vi "Xijk.vi"() -> ()   [LabVIEW 2010]
uses:
  Type Def/filepath.ctl
  Type Def/event.ctl
  Type Def/axis_parameters.ctl
  Type Def/color_parameters.ctl
  Type Def/save_cluster.ctl
  Type Def/configuration_cluster.ctl
  Type Def/search_parameters.ctl
  Type Def/spectra_parameters.ctl
  Type Def/settings.ctl
  Type Def/spectrum_table_control.ctl
  Type Def/xijk_cluster.ctl
  Type Def/control_references_cluster.ctl
  <vilib>/Utility/miscctls.llb/LVPointTypeDef.ctl
  <vilib>/Utility/xml.llb/Write to XML File(string).vi
  subVI/xijk_automatic_read_and_guess.lvlib
  subVI/xijk_select_best_filter.lvlib
  subVI/xijk_combined_file.lvlib
panel:
  in  "Settings":T1={"search parameters"={"Paths"={"Path: Excitation filters"=path "", "Path: Dicroic filters"=path "", "Path: Emission filters"=path "", "Path reget"=path ""}, "table excitation"=[], "table dicroics"=[], "table emission"=[], "Integers"={"Select result number"=1}, "boolean selector array"=[], "table for calculation automagic"=[]}, "output cluster"={"Booleans"={"Unknown detector"=FALSE, "Dual band filters"=FALSE, "Dual emission by cubes"=FALSE, "FRET"=FALSE}, "Integers"={"Light source"=0, "Number of fluorophores"=0, "Wavelength of laser (nm) 1"=0, "Broadness of laser (nm) 1"=0.0, "Wavelength of laser (nm) 2"=0, "Broadness of laser (nm) 2"=0.0, "Template"=1}, "Doubles"={"Molar extinction 1"=1.0, "Molar extinction 2"=1.0, "Quantum efficiency 1"=1.0, "Quantum efficiency 2"=1.0}}, "output cluster 2"={"Excitation filter 1"=path "", "Dichroic filter 1"=path "", "Emission filter 1"=path "", "Excitation filter 2"=path "", "Dichroic filter 2"=path "", "Emission filter 2"=path "", "Extra em filter 1"=path "", "Extra em filter 2"=path "", "Light source file"=path "", "Fluorophore absorption 1"=path "", "Fluorophore emission 1"=path "", "Fluorophore absorption 2"=path "", "Fluorophore emission 2"=path "", "Detector"=path ""}, "cluster de sortie"={"Excitation filter_x"=[], "Excitation filter_y"=[], "Dichroic filter_x"=[], "Dichroic filter_y"=[], "Emission filter_x"=[], "Emission filter_y"=[], "Excitation filter_x 2"=[], "Excitation filter_y 2"=[], "Dichroic filter_x 2"=[], "Dichroic filter_y 2"=[], "Emission filter_x 2"=[], "Emission filter_y 2"=[], "Extra em filter_x 1"=[], "Extra em filter_y 1"=[], "Extra em filter_x 1"=[], "Extra em filter_y 2"=[], "Light source_x"=[], "Light source_y"=[], "Detector_x"=[], "Detector_y"=[], "Fluorophore absorption_x"=[], "Fluorophore absorption_y"=[], "Fluorophore emission_x"=[], "Fluorophore emission_y"=[], "Fluorophore absorption_x 2"=[], "Fluorophore absorption_y 2"=[], "Fluorophore emission_x 2"=[], "Fluorophore emission_y 2"=[], "laser_x"=[], "laser_y"=[], "laser_x 2"=[], "laser_y 2"=[], "quantum efficiency factor 1"=0.0, "quantum efficiency factor 2"=0.0, "lamp scaling factor"=0.0}, "Xijk output cluster"={"Xijk 111"=0.0, "Xijk 112"=0.0, "Xijk 121"=0.0, "Xijk 122"=0.0, "Xijk 211"=0.0, "Xijk 212"=0.0, "Xijk 221"=0.0, "Xijk 222"=0.0, "Eijk 111"=0.0, "Eijk 112"=0.0, "Eijk 121"=0.0, "Eijk 122"=0.0, "Eijk 211"=0.0, "Eijk 212"=0.0, "Eijk 221"=0.0, "Eijk 222"=0.0}, "GUI configuration"={"axes in"={"min x-axis excitation"=300, "max x-axis excitation"=800, "min x-axis emission"=300, "max x-axis emission"=800, "precision of results"=2}, "plot colors in"={"Lanscape Portrait"=FALSE, "Plot logarithmic"=FALSE, "Ex/Em filters double"=FALSE, "Line colors"=[16734569, 56375, 16711916, 5896447, 16448250, 56375]}}, "references"={"Excitation filter 1 ref"=refnum, "Dichroic filter 1 ref"=refnum, "Emission filter 1 ref"=refnum, "Excitation filter 2 ref"=refnum, "Dichroic filter 2 ref"=refnum, "Emission filter 2 ref"=refnum, "Extra em filter 1 ref"=refnum, "Extra em filter 2 ref"=refnum, "Light source file ref"=refnum, "Fluorophore absorption 1 ref"=refnum, "Fluorophore emission 1 ref"=refnum, "Fluorophore absorption 2 ref"=refnum, "Fluorophore emission 2 ref"=refnum, "Detector ref"=refnum}} {"GUI configuration"."axes in"."precision of results" max=8 step=1}
  out "Filter cube 1 excitation":cluster{"Y":dbl[], "Y":dbl[]}[](graph)
  in  "save cluster":T11={"Project name"="", "configuration"={"axes in"={"min x-axis excitation"=0, "max x-axis excitation"=0, "min x-axis emission"=0, "max x-axis emission"=0, "precision of results"=2}, "plot colors in"={"Lanscape Portrait"=FALSE, "Plot logarithmic"=FALSE, "Ex/Em filters double"=FALSE, "Line colors"=[]}}, "search paths in"={"Paths"={"Path: Excitation filters"=path "", "Path: Dicroic filters"=path "", "Path: Emission filters"=path "", "Path reget"=path ""}, "table excitation"=[], "table dicroics"=[], "table emission"=[], "Integers"={"Select result number"=0}, "boolean selector array"=[], "table for calculation automagic"=[]}, "spectra parameters in"={"Booleans"={"Unknown detector"=FALSE, "Dual band filters"=FALSE, "Dual emission by cubes"=FALSE, "FRET"=FALSE}, "Integers"={"Light source"=0, "Number of fluorophores"=0, "Wavelength of laser (nm) 1"=0, "Broadness of laser (nm) 1"=0.0, "Wavelength of laser (nm) 2"=0, "Broadness of laser (nm) 2"=0.0, "Template"=0}, "Doubles"={"Molar extinction 1"=0.0, "Molar extinction 2"=0.0, "Quantum efficiency 1"=0.0, "Quantum efficiency 2"=0.0}}, "filepaths in"={"Excitation filter 1"=path "", "Dichroic filter 1"=path "", "Emission filter 1"=path "", "Excitation filter 2"=path "", "Dichroic filter 2"=path "", "Emission filter 2"=path "", "Extra em filter 1"=path "", "Extra em filter 2"=path "", "Light source file"=path "", "Fluorophore absorption 1"=path "", "Fluorophore emission 1"=path "", "Fluorophore absorption 2"=path "", "Fluorophore emission 2"=path "", "Detector"=path ""}} {"configuration"."axes in"."precision of results" max=8 step=1}
  in  "start path":path=path ""
  in  "Tabs wizard":T12(tab)
  in  "stop wizard 1":bool
  in  "Page 0. Next":bool
  in  "Page 1. Previous":bool
  in  "stop wizard 2":bool
  in  "Page 1. Next":bool
  in  "stop wizard 3":bool
  in  "Page 2. Previous":bool
  in  "Page 2. Next":bool
  in  "stop wizard 4":bool
  in  "Page 3. Previous":bool
  in  "Page 3. Next":bool
  in  "stop wizard 5":bool
  in  "Page 4. Previous":bool
  in  "Page 4. Next":bool
  in  "stop wizard 6":bool
  in  "Page 5. Previous":bool
  in  "Page 5. Next":bool
  in  "stop wizard 7":bool
  in  "Page 6. Previous":bool
  in  "Page 6. Next":bool
  in  "stop wizard 8":bool
  in  "Page 7. Previous":bool
  in  "Page 7. Next":bool
  in  "stop wizard 9":bool
  in  "Page 8. Previous":bool
  in  "Page 8. Next":bool
  in  "stop wizard 10":bool
  in  "Page 9. Previous":bool
  in  "Page 9. Next":bool
  in  "stop wizard 11":bool
  in  "Page 10. Previous":bool
  in  "Page 10. Next":bool
  in  "stop wizard 12":bool
  in  "Page 11. Previous":bool
  in  "Page 11. Next":bool
  in  "stop wizard 13":bool
  in  "Page 12. Previous":bool
  out "start time":u32
  out "Table of settings":path[](array[path])
  out "light source value":u16
  out "hide detector box?":bool
  in  "width":u8[][](array[numeric])=[[1, 1, 2, 1, 1, 1], [1, 1, 2, 1, 1, 1], [1, 1, 1, 2, 1, 1], [1, 1, 1, 2, 1, 1], [0, 0, 0, 0, 0, 0], [0, 0, 0, 0, 0, 0]]
  in  "style":u8[][](array[numeric])=[[0, 0, 0, 2, 0, 2], [0, 0, 0, 2, 0, 2], [0, 0, 2, 0, 0, 2], [0, 0, 2, 0, 0, 2], [0, 0, 0, 0, 0, 0], [0, 0, 0, 0, 0, 0]]
  out "Filter cube 2 excitation":cluster{"Y":dbl[], "Y":dbl[]}[](graph)
  out "Filter cube 2 emission":cluster{"Y":dbl[], "Y":dbl[]}[](graph)
  out "Filter cube 1 emission":cluster{"Y":dbl[], "Y":dbl[]}[](graph)
  in  "Tab results":T13(tab)
  out "Eijk 111":sgl format="%.2f"
  out "Eijk 121":sgl format="%.2f"
  out "Eijk 122":sgl format="%.2f"
  out "Eijk 112":sgl format="%.2f"
  out "Eijk 212":sgl format="%.2f"
  out "Eijk 211":sgl format="%.2f"
  out "Eijk 222":sgl format="%.2f"
  out "Eijk 221":sgl format="%.2f"
  in  "Help Eijk":bool
  out "Xijk 111":sgl format="%.2f"
  out "Xijk 121":sgl format="%.2f"
  out "Xijk 122":sgl format="%.2f"
  out "Xijk 112":sgl format="%.2f"
  out "Xijk 212":sgl format="%.2f"
  out "Xijk 211":sgl format="%.2f"
  out "Xijk 222":sgl format="%.2f"
  out "Xijk 221":sgl format="%.2f"
  in  "Help Xijk":bool
  in  "Help Others":bool
  out "% Absorption":dbl format="%#_3g"
  out "% Emission":dbl format="%#_3g"
  out "excitation light bleed through":dbl caption="% Exc. bleed through" format="%#_3g"
  out "excitation light bleed through 2":dbl caption="% Exc. bleed through" format="%#_3g"
  out "% Emission":dbl format="%#_3g"
  out "% Absorption":dbl format="%#_3g"
  out "Spectral overlap efficiency":dbl format="%#_3g"
  out "% Green emission in red channel":dbl format="%#_3g"
  out "% Red emission in green channel":dbl format="%#_3g"
  in  "Help Config":bool
  in  "axes in":T8={"min x-axis excitation"=300, "max x-axis excitation"=800, "min x-axis emission"=300, "max x-axis emission"=800, "precision of results"=2} caption="Range axes" {"precision of results" max=8 step=1}
  in  "plot colors in":T9={"Lanscape Portrait"=FALSE, "Plot logarithmic"=FALSE, "Ex/Em filters double"=FALSE, "Line colors"=[16734569, 56375, 16711916, 5896447, 16448250, 56375]} caption="Plot"
  in  "Select result number":u32 caption="Select result n°"
  in  "Help Automatized":bool
  in  "Path: Emission filters":path
  in  "2. Emission":bool
  in  "2. Dichroic":bool
  in  "2. Excitation":bool
  in  "1. Emission":bool
  in  "1. Dichroic":bool
  in  "1. Excitation":bool
  in  "Path: Excitation filters":path
  in  "fast search?":bool=TRUE
  in  "Path reget":path
  in  "Path: Dicroic filters":path
  out "Result template":enum32{"0", "1", "2", "3", "4", "5", "6", "7"}(tab)
  in  "Help Templates":bool
  in  "Help Templates 3":bool
  in  "Help Templates 4":bool
  in  "Help Templates 5":bool
  in  "Help Templates 6":bool
  in  "Help Templates 7":bool
  in  "Help Templates 8":bool
  in  "Help Templates 9":bool
  in  "Select template":u16(ring) items=["Personal", "Basic single fluorophore", "Single excitation dual emission", "Single excitation dual detection", "Single excitation FRET dual emission", "Single excitation FRET dual detection", "Dual excitation dual emission", "Dual excitation dual detection"]
  in  "Help Examples":bool
  in  "Examples":u8(ring) items=["none", "ACR", "CFP", "CFP-YFP", "DAPI", "eGFP", "eGFP Bodipy R6G", "eGFP-AO", "eGFP-Ca-TM1", "eGFP-Ca-TM2", "eGFP-Calcium Crimson", "eGFP-CaSiR-1", "eGFP-Fura Red", "eGFP-ICPBC", "eGFP-KFCA", "FITC", "FITC-TxRed", "Rhodamine 6G", "YFP"]
  in  "button:create_function":bool caption="Create custom filter"
  in  "button:image_to_text":bool caption="Convert image to text file"
  in  "Tabs parameters":T14(tab)
  in  "Help Fluorophore":bool
  out "fluorophores hide box":bool
  out "Brightness 2":sgl caption="Brightness"
  out "Brightness":sgl
  in  "Quantum efficiency 2":sgl=1.0 min=0
  in  "Quantum efficiency 1":sgl=1.0 min=0
  in  "Molar extinction 2":sgl=1.0 min=0
  in  "Fluorophore absorption 2":path
  in  "Fluorophore emission 2":path
  in  "Molar extinction 1":sgl=1.0 min=0
  in  "Fluorophore absorption":path
  in  "Fluorophore emission":path
  in  "FRET":bool
  in  "Number of fluorophores":u16(ring)=1 items=["1", "2"]
  in  "Light source":u16(ring) items=["Load spectrum", "1 Gaussian", "2 Gaussian"]
  out "Tab Control":enum32{"Page 1", "Page 2"}(tab)
  in  "Light source file":path
  in  "Help Exciter 2":bool
  out "laser hide box":bool
  in  "Wavelength of laser (nm) 1":u16=400 min=1 max=1200
  in  "Broadness of laser (nm) 1":sgl=1.0 min=1 max=1200
  in  "Wavelength of laser (nm) 2":u16=500 min=1 max=1200
  in  "Broadness of laser (nm) 2":sgl=1.0 min=1 max=1200
  in  "Help Exciter":bool
  in  "Excitation filter 1":path
  in  "Extra em filter 2":path
  in  "Extra em filter 1":path
  in  "Dichroic filter 2":path
  in  "Dichroic filter 1":path
  in  "Emission filter 1":path
  in  "Emission filter 2":path
  in  "Excitation filter 2":path
  in  "Help Filters":bool
  out "detector hide box":bool
  in  "Dual band filters":bool
  in  "Unknown detector":bool=TRUE
  in  "Detector":path
  in  "Dual emission by cubes":bool=TRUE
  in  "Help Detector":bool
  in  "error in":errorcluster
  in  "task":T15=enum."Update filter names"
  in  "filepaths in":T4
  in  "Tab Buttons":enum32{"Page 2"}(tab)
  in  "Button load":bool
  in  "Button save":bool
  in  "Button automagic":bool
  in  "Button stop":bool
  in  "Button reset":bool
  in  "Button export":bool
  in  "Button Help":bool
  in  "Help pictograms":bool
  in  "Tab Header":enum32{"Page 2"}(tab)
  in  "Project name":string
  out "Runtime":dbl format="%.2f"
  out "Busy":bool
  out "Slide":dbl(slide) scale=0.0..1.0
  # "Xijk tool"
  # "Developed by: Marcel van 't Hoff & Martin Oheim"
  # "Dichroic"
  # "Ex/Em filter"
  # "Fluorophore 1"
  # "Fluorophore 2"
  # "Laser /\nextra Em filter"
  # "Dichroic"
  # "Ex/Em filter"
  # "Fluorophore 1"
  # "Fluorophore 2"
  # "Laser /\nextra Em filter"
  # "Xijk"
  # "Xijk is a mathematical indicator for the quality of separation of two fluorophores in the microscopy by the choice of filters.\n\nXijk is calculated by the effective spectral excitation and emission, Eijk, for a specific light source (i), on a specific fluorophore (j), detected on a specific channel (k).\nThe unique Eijk divided by the sum of all Eijk gives the unique Xijk. The Xijk for each channel ranges from 0 to 1, where in the spefic channels for your setting you want to have the maximal separation. \n\nXijk gives a qualitive indication\nEijk gives a quantitive indication \n\n\nThe Wizard will start and guide you through the initial steps"
  # "Step I"
  # "First you will need to select the right fluorophores here on the left. Select the right absorption and emission spectra of the two dyes.\n\nFluorophore 1 should be the most blue dye.\nFluorophore 2 should be the most red dye.\n\n- Select first the right amount of dyes. \n\n- Fill in the molar extinction\n\n- Fill in the quantum efficiency"
  # "Step II"
  # "Select the right light source, matching your experiment. \nThe broadness can be changed, but a value of 2 nm is rather normal."
  # "Step III"
  # "Select here the excitation filter, dicroic and emission filter. Each specific for the corresponding dyes.\nExtra emission filters can be selected\n\n- Select the excitation filter that matches your light source.\n\n- Select the dichroic such that most excitation is reflected and most emission light from the fluorophores is transmitted\n\n- Select the emission filter such that most emission light is transmitted, but such that the emission is selective this fluorophore and has few overlap with the other dye."
  # "Step IV"
  # "Select here your detection spectrum.\nIn case of unknown detector spectrum, a 100% spectrum is used.\n\n- Dual emission detection is often done by changing the filter cubes for each fluorophore. \n  Dual detection separates the emission light with the second dichroic into two channels. \n\n- By notch filtering, emission light is selected by removing the excitation light by a narrow band-block filter. Which can be practical for experiments where the Stoke's shift is small."
  # "Step V"
  # "Here can be selected for a specific template. The schemes represent the different settings. After selecting a template, the variables can not be changed anymore. Use Personal for your own settings.\n\n- Selecting a template has the advantage you can not make mistakes and have the interesting Eijk and Xijk automatically selected."
  # "Step VI"
  # "Here can be selected for a small collection of examples."
  # "Step VII"
  # "Here is one of the two most interesting pages. Here the values of each Eijk is calculated. Depending on the configuration or template, the Eijk are highlighted or not.\n\n- Example 1: Eijk 111 gives the integral upon excitation with light source (1xx), the emitted emission of fluorophore (x1x) detected in channel (xx1). A high value indicates that upon the right excitation, the right fluorophores emission is detected in the right channel.\n\n- Example 2: Eijk 121 gives upon excitation of light source (1xx), the emitted emission of fluorophore (x2x) detected in channel (xx1). A low value indicates that you do not detect fluorescence of the second dye in the first channel upon excitation of the first fluorophore."
  # "Step VIII"
  # "Following the Eijk values, the Xijk values are shown here."
  # "Step IX"
  # "Here is shown how effectively the fluorophores are excited and how much of the emitted fluororescence is captured."
  # "Step X"
  # "In this page you can configure a few settings. The ranges of the axes can be changed and also the colors of the curves.\nNext, the precision of the results can be changed."
  # "Step XI"
  # "The last step, but maybe the most practical.\nIn this step you can select the directory that contains the excitation, dicroic and emission filters. The program searches for all filters in this folder.\nSelect for which parameters you would like to optimize.\n\nBe cautious. The time to calculate scales with the number of filters to the power of number of optimization. \n\nWhen this is started, it automatically asked where to save the file with results.\n\nLater you can select which result number you would like to have from a saved table."
  # "Step XII"
  # "Here are the controls.\n\n\n            Reset                             Save\n\n\n\n            Stop                              Load\n\n\n\n            Export                            Help\n\n\n\n            Find                               Reget"
  # "Dichroic"
  # "Ex/Em filter"
  # "Fluorophore 1"
  # "Fluorophore 2"
  # "Laser /\nextra Em filter"
  # "Optimize for:"
  # "?"
  # "?"
  # "?"
  # "EX1"
  # "1"
  # "D1"
  # "EM1"
  # "1"
  # "1"
  # "EX2"
  # "EM2"
  # "D2"
  # "EX1"
  # "1"
  # "2"
  # "D1"
  # "EM1"
  # "2"
  # "1"
  # "1"
  # "EX2"
  # "EM2"
  # "M"
  # "EX1"
  # "1"
  # "2"
  # "D1"
  # "D2"
  # "EM1"
  # "2"
  # "1"
  # "1"
  # "EX2"
  # "EM2"
  # "D2"
  # "FRET"
  # "EX1"
  # "1"
  # "2"
  # "D1"
  # "EM1"
  # "2"
  # "1"
  # "1"
  # "EX2"
  # "EM2"
  # "M"
  # "FRET"
  # "EX1"
  # "1"
  # "2"
  # "D1"
  # "D2"
  # "EM1"
  # "2"
  # "1"
  # "1"
  # "EX2"
  # "EM2"
  # "D2"
  # "EX1"
  # "1"
  # "2"
  # "D1"
  # "EM1"
  # "2"
  # "1"
  # "2"
  # "1"
  # "EM2"
  # "M"
  # "EX1"
  # "1"
  # "2"
  # "D1"
  # "D2"
  # "EM1"
  # "1"
  # "2"
  # "1"
  # "2"
  # "1"
  # "ABS"
  # "1"
  # "EM"
  # "e"
  # "QE"
  # "2"
  # "ABS"
  # "2"
  # "EM"
  # "e"
  # "QE"
  # "Lamp"
  # "1"
  # "2"
  # "Center (nm)"
  # "FWHM (nm)"
  # "Center (nm)"
  # "FWHM (nm)"
  # "2"
  # "1"
  # "EX1"
  # "D1"
  # "EM1"
  # "EX2"
  # "D2"
  # "EM2"
  # "Extra EM1"
  # "Extra EM2"
  # "DET"
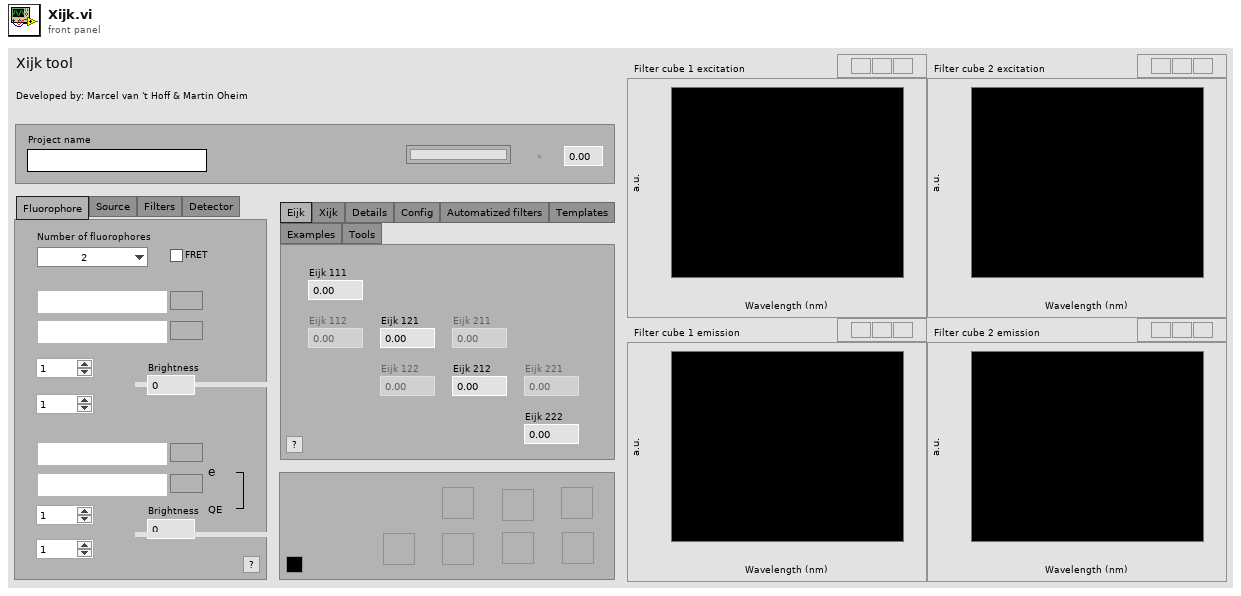
[diagram p1: front panel]
types:
  T1 = typedef "settings.ctl" = cluster{"search parameters":T2, "output cluster":T3, "output cluster 2":T4, "cluster de sortie":T5, "Xijk output cluster":T6, "GUI configuration":T7, "references":T10}
  T2 = typedef "search_parameters.ctl" = cluster{"Paths":cluster{"Path: Excitation filters":path, "Path: Dicroic filters":path, "Path: Emission filters":path, "Path reget":path}, "table excitation":path[], "table dicroics":path[], "table emission":path[], "Integers":cluster{"Select result number":u32}, "boolean selector array":bool[], "table for calculation automagic":i32[]}
  T3 = typedef "spectra_parameters.ctl" = cluster{"Booleans":cluster{"Unknown detector":bool, "Dual band filters":bool, "Dual emission by cubes":bool, "FRET":bool}, "Integers":cluster{"Light source":u16, "Number of fluorophores":u16, "Wavelength of laser (nm) 1":u16, "Broadness of laser (nm) 1":sgl, "Wavelength of laser (nm) 2":u16, "Broadness of laser (nm) 2":sgl, "Template":u16}, "Doubles":cluster{"Molar extinction 1":sgl, "Molar extinction 2":sgl, "Quantum efficiency 1":sgl, "Quantum efficiency 2":sgl}}
  T4 = typedef "filepath.ctl" = cluster{"Excitation filter 1":path, "Dichroic filter 1":path, "Emission filter 1":path, "Excitation filter 2":path, "Dichroic filter 2":path, "Emission filter 2":path, "Extra em filter 1":path, "Extra em filter 2":path, "Light source file":path, "Fluorophore absorption 1":path, "Fluorophore emission 1":path, "Fluorophore absorption 2":path, "Fluorophore emission 2":path, "Detector":path}
  T5 = typedef "spectrum_table_control.ctl" = cluster{"Excitation filter_x":i16[], "Excitation filter_y":sgl[], "Dichroic filter_x":i16[], "Dichroic filter_y":sgl[], "Emission filter_x":i16[], "Emission filter_y":sgl[], "Excitation filter_x 2":i16[], "Excitation filter_y 2":sgl[], "Dichroic filter_x 2":i16[], "Dichroic filter_y 2":sgl[], "Emission filter_x 2":i16[], "Emission filter_y 2":sgl[], "Extra em filter_x 1":i16[], "Extra em filter_y 1":sgl[], "Extra em filter_x 1":i16[], "Extra em filter_y 2":sgl[], "Light source_x":i16[], "Light source_y":sgl[], "Detector_x":i16[], "Detector_y":sgl[], "Fluorophore absorption_x":i16[], "Fluorophore absorption_y":sgl[], "Fluorophore emission_x":i16[], "Fluorophore emission_y":sgl[], "Fluorophore absorption_x 2":i16[], "Fluorophore absorption_y 2":sgl[], "Fluorophore emission_x 2":i16[], "Fluorophore emission_y 2":sgl[], "laser_x":i16[], "laser_y":sgl[], "laser_x 2":i16[], "laser_y 2":sgl[], "quantum efficiency factor 1":sgl, "quantum efficiency factor 2":sgl, "lamp scaling factor":sgl}
  T6 = typedef "xijk_cluster.ctl" = cluster{"Xijk 111":sgl, "Xijk 112":sgl, "Xijk 121":sgl, "Xijk 122":sgl, "Xijk 211":sgl, "Xijk 212":sgl, "Xijk 221":sgl, "Xijk 222":sgl, "Eijk 111":sgl, "Eijk 112":sgl, "Eijk 121":sgl, "Eijk 122":sgl, "Eijk 211":sgl, "Eijk 212":sgl, "Eijk 221":sgl, "Eijk 222":sgl}
  T7 = typedef "configuration_cluster.ctl" = cluster{"axes in":T8, "plot colors in":T9}
  T8 = typedef "axis_parameters.ctl" = cluster{"min x-axis excitation":u16, "max x-axis excitation":u16, "min x-axis emission":u16, "max x-axis emission":u16, "precision of results":u8}
  T9 = typedef "color_parameters.ctl" = cluster{"Lanscape Portrait":bool, "Plot logarithmic":bool, "Ex/Em filters double":bool, "Line colors":u32[]}
  T10 = typedef "control_references_cluster.ctl" = cluster{"Excitation filter 1 ref":refnum<vi>, "Dichroic filter 1 ref":refnum<vi>, "Emission filter 1 ref":refnum<vi>, "Excitation filter 2 ref":refnum<vi>, "Dichroic filter 2 ref":refnum<vi>, "Emission filter 2 ref":refnum<vi>, "Extra em filter 1 ref":refnum<vi>, "Extra em filter 2 ref":refnum<vi>, "Light source file ref":refnum<vi>, "Fluorophore absorption 1 ref":refnum<vi>, "Fluorophore emission 1 ref":refnum<vi>, "Fluorophore absorption 2 ref":refnum<vi>, "Fluorophore emission 2 ref":refnum<vi>, "Detector ref":refnum<vi>}
  T11 = typedef "save_cluster.ctl" = cluster{"Project name":string, "configuration":T7, "search paths in":T2, "spectra parameters in":T3, "filepaths in":T4}
  T12 = enum32{"Page 0", "Page 1", "Page 2", "Page 3", "Page 4", "Page 5", "Page 6", "Page 7", "Page 8", "Page 9", "Page 10", "Page 11", "Page 12"}
  T13 = enum32{"Eijk", "Xijk", "Details", "Config", "Automatized filters", "Templates", "Examples", "Tools"}
  T14 = enum32{"Fluorophore", "Source", "Filters", "Detector"}
  T15 = typedef "event.ctl" = enum16{"Initialise parameters", "Initialise paths", "Execute", "Hide detector", "Light source selection", "Get example list", "Set Example", "Change portrait / landscape", "Dual band cube", "Save to file", "Load from file", "Set filepaths to boxes", "1 or 2 fluorophore selection", "Update configurations", "Update template", "Calculate other values", "Update filter names", "Shutdown", "Shutdown - hard exit", "Search in filters - set parameters", "Search in filters - search", "Search in filters - get xijk", "Search in filters - reget", "Optimize - Sort table", "Get path from search", "Calculate Xijk", "Get spectra from files", "Create graphs", "Reset variables", "Tools - convert image to text", "Tools - create function", "Help - open", "Help - close", "Help - next", "Help - previous", "Help - select menu", "Export data"}
  T16 = typedef "LVPointTypeDef.ctl" = cluster{"Horizontal":i16, "Vertical":i16}
  T17 = cluster{"min x-axis excitation":dbl, "max x-axis excitation":dbl, "min x-axis emission":dbl, "max x-axis emission":dbl, "precision of results":dbl}
  T18 = enum8{"Enabled", "Disabled", "Disabled and Grayed Out"}[]
  T19 = enum8{"Enabled", "Disabled", "Disabled and Grayed Out"}
  T20 = typedef "LVRectTypeDef.ctl" = cluster{"left":i16, "top":i16, "right":i16, "bottom":i16}
  T21 = enum32{"invalid app kind", "Development System", "Run Time System", "Student Edition", "Embedded LabVIEW", "Evaluation", "Custom"}
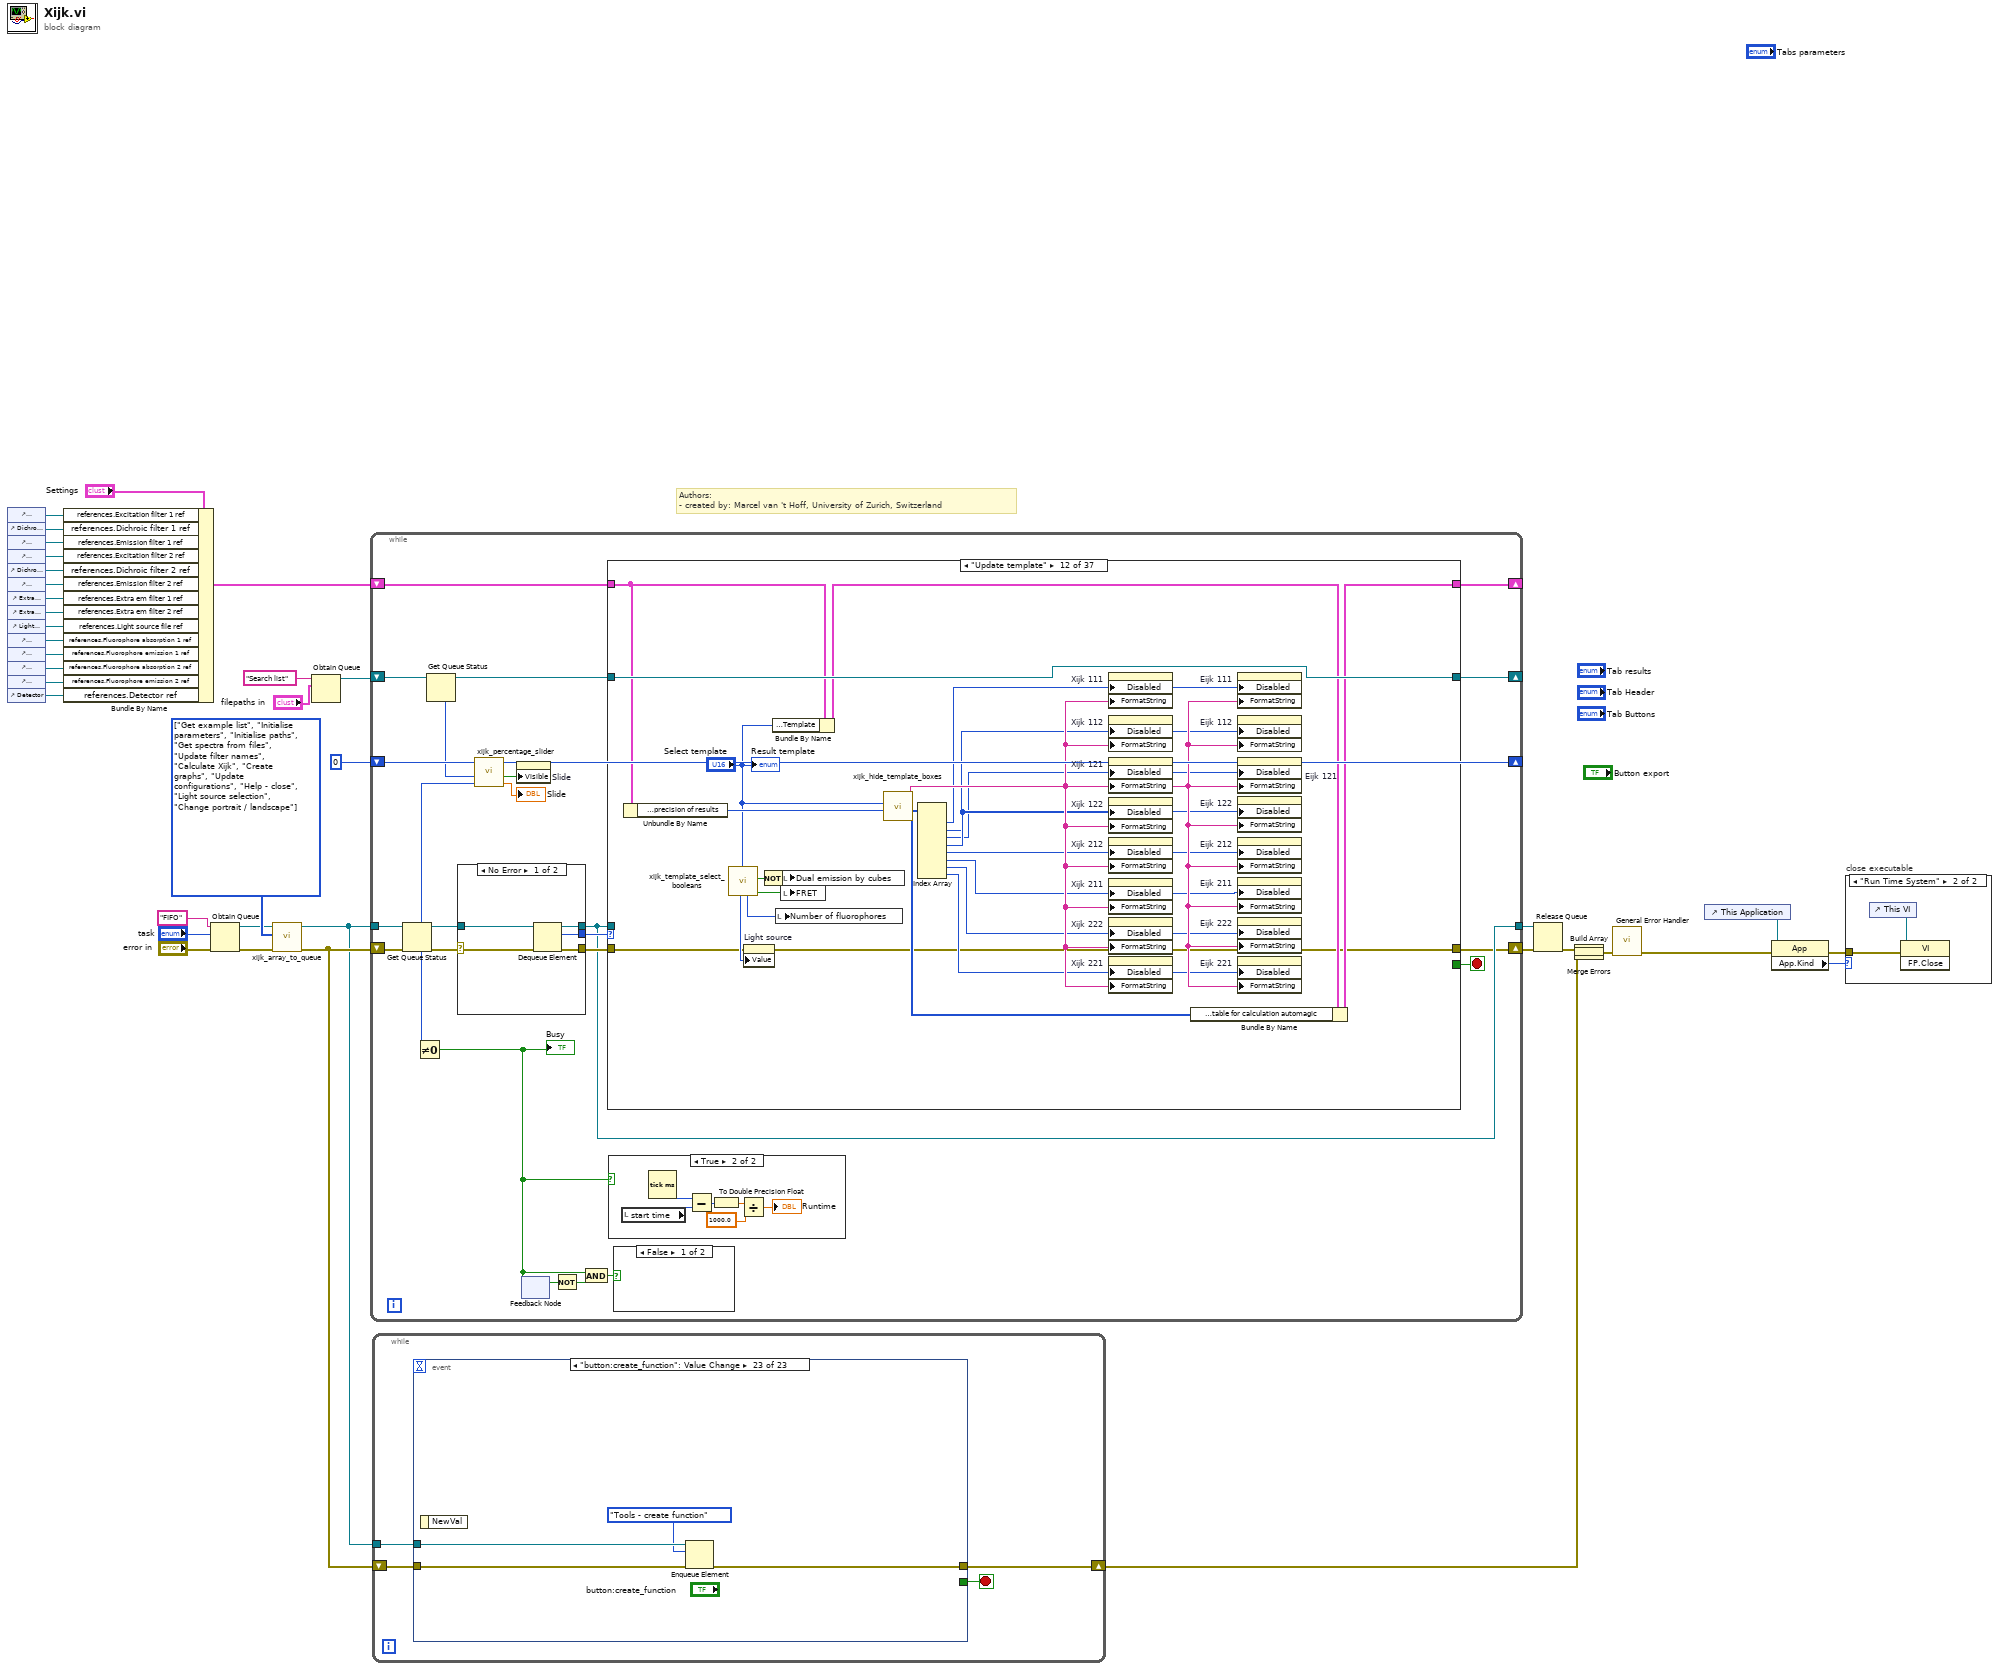
[diagram p0: block diagram]
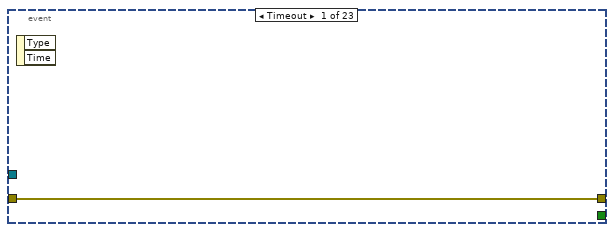
[diagram p3: hidden frame]
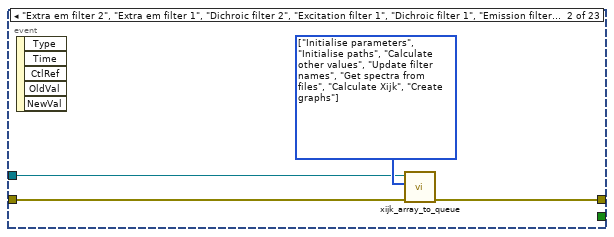
[diagram p4: hidden frame]
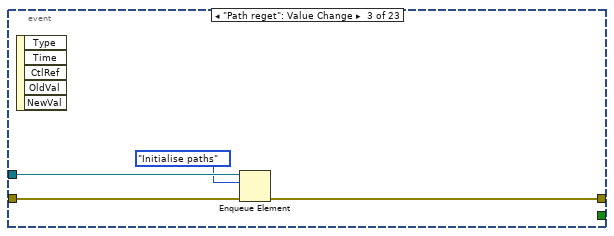
[diagram p5: hidden frame]
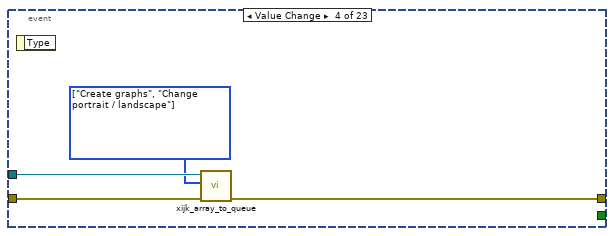
[diagram p6: hidden frame]
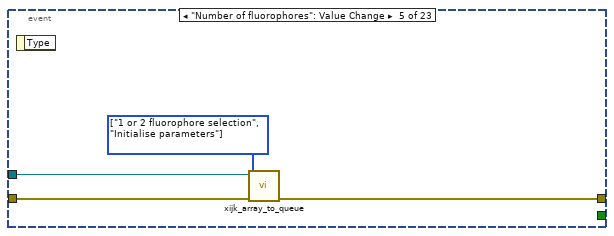
[diagram p7: hidden frame]
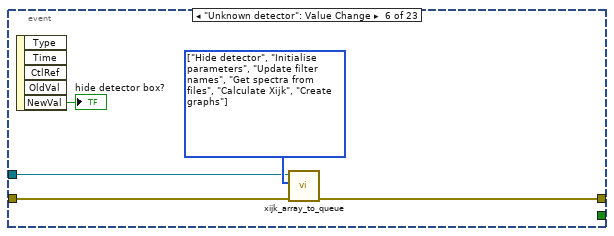
[diagram p8: hidden frame]
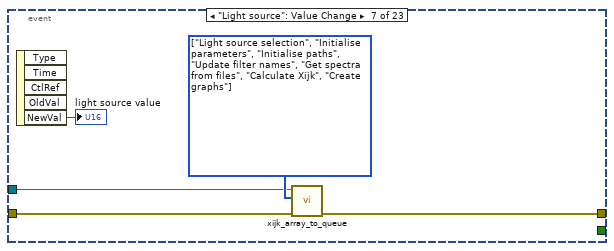
[diagram p9: hidden frame]
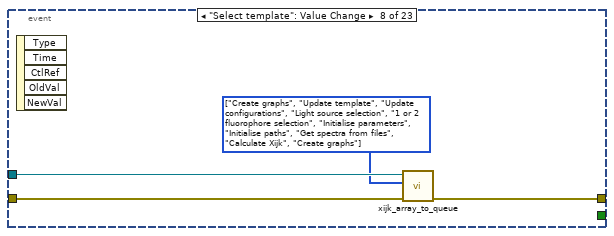
[diagram p10: hidden frame]
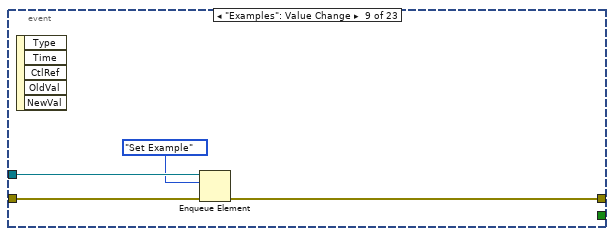
[diagram p11: hidden frame]
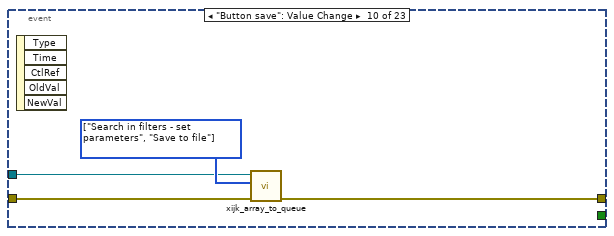
[diagram p12: hidden frame]
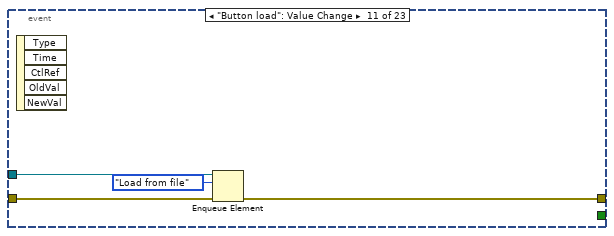
[diagram p13: hidden frame]
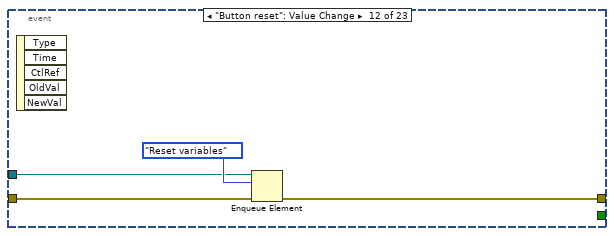
[diagram p14: hidden frame]
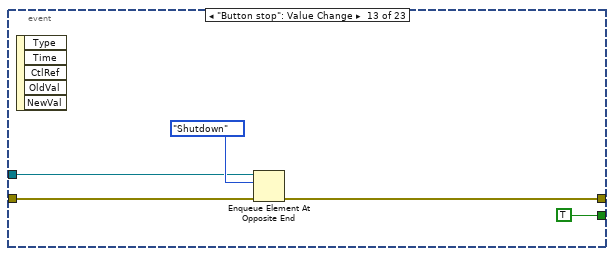
[diagram p15: hidden frame]
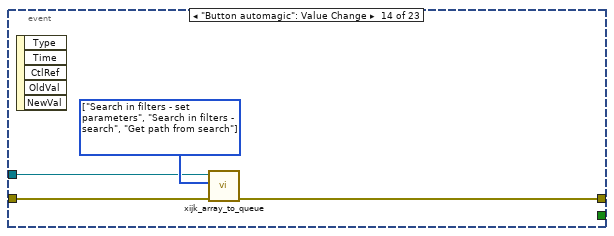
[diagram p16: hidden frame]
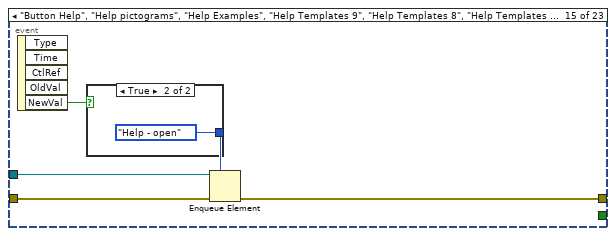
[diagram p17: hidden frame]
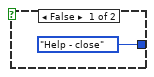
[diagram p18: hidden frame]
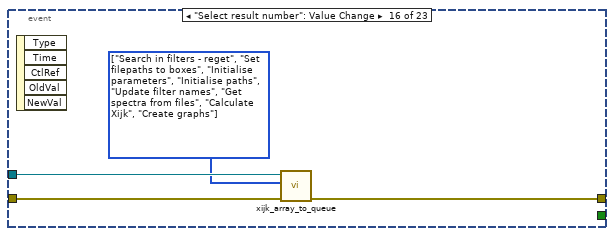
[diagram p19: hidden frame]
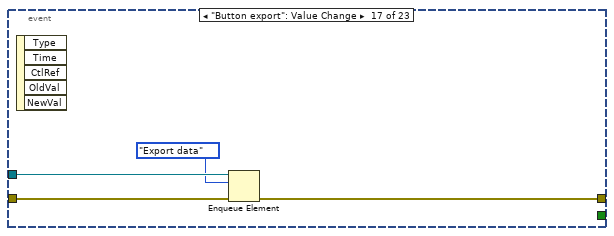
[diagram p20: hidden frame]
diagram:
  w29 = T15[] [enum."Get example list", enum."Initialise parameters", enum."Initialise paths", enum."Get spectra from files", enum."Update filter names", enum."Calculate Xijk", enum."Create graphs", enum."Update configurations", enum."Help - close", enum."Light source selection", enum."Change portrait / landscape"] items=["Initialise parameters", "Initialise paths", "Execute", "Hide detector", "Light source selection", "Get example list", "Set Example", "Change portrait / landscape", "Dual band cube", "Save to file", "Load from file", "Set filepaths to boxes", "1 or 2 fluorophore selection", "Update configurations", "Update template", "Calculate other values", "Update filter names", "Shutdown", "Shutdown - hard exit", "Search in filters - set parameters", "Search in filters - search", "Search in filters - get xijk", "Search in filters - reget", "Optimize - Sort table", "Get path from search", "Calculate Xijk", "Get spectra from files", "Create graphs", "Reset variables", "Tools - convert image to text", "Tools - create function", "Help - open", "Help - close", "Help - next", "Help - previous", "Help - select menu", "Export data"]
  # "Authors: \n- created by: Marcel van 't Hoff, University of Zurich, Switzerland"
  n1 = control-ref of="Excitation filter 1"() -> (w17:refnum<vi>)
  n2 = control-ref of="Dichroic filter 1"() -> (w16:refnum<vi>)
  n3 = control-ref of="Emission filter 1"() -> (w15:refnum<vi>)
  n4 = control-ref of="Excitation filter 2"() -> (w14:refnum<vi>)
  n5 = control-ref of="Dichroic filter 2"() -> (w13:refnum<vi>)
  n6 = control-ref of="Emission filter 2"() -> (w12:refnum<vi>)
  n7 = control-ref of="Extra em filter 1"() -> (w11:refnum<vi>)
  n8 = control-ref of="Extra em filter 2"() -> (w10:refnum<vi>)
  n9 = control-ref of="Light source file"() -> (w9:refnum<vi>)
  n10 = control-ref of="Fluorophore absorption"() -> (w8:refnum<vi>)
  n11 = control-ref of="Fluorophore emission"() -> (w7:refnum<vi>)
  n12 = control-ref of="Fluorophore absorption 2"() -> (w6:refnum<vi>)
  n13 = control-ref of="Fluorophore emission 2"() -> (w5:refnum<vi>)
  n14 = control-ref of="Detector"() -> (w4:refnum<vi>)
  n15 = Bundle By Name(cluster="Settings", "references.Excitation filter 1 ref"=w17, "references.Dichroic filter 1 ref"=w16, "references.Emission filter 1 ref"=w15, "references.Excitation filter 2 ref"=w14, "references.Dichroic filter 2 ref"=w13, "references.Emission filter 2 ref"=w12, "references.Extra em filter 1 ref"=w11, "references.Extra em filter 2 ref"=w10, "references.Light source file ref"=w9, "references.Fluorophore absorption 1 ref"=w8, "references.Fluorophore emission 1 ref"=w7, "references.Fluorophore absorption 2 ref"=w6, "references.Fluorophore emission 2 ref"=w5, "references.Detector ref"=w4) -> (w1:T1)
  n16 = Obtain Queue(name (unnamed)="FIFO", element data type="task", error in (no error)="error in") -> (queue out=w27:refnum<queue>, error out=w31:errorcluster)  [unwired: 2 in, 1 out]
  n17 = call "xijk_array_to_queue.vi"("error in"=w31, "array in"=w29, "queue in"=w27) -> ("error out"=w30:errorcluster, "queue out"=w26:refnum<queue>)  [unwired: 7 in]
  n18 = Obtain Queue(name (unnamed)="Search list", element data type="filepaths in") -> (queue out=w23:refnum<queue>)  [unwired: 3 in, 2 out]
  n19 = while {
    tunnel: w26 -> [w54]
    tunnel: [w60] -> w36
    shift-right: [w58] -> w34
    shift-left: w30 -> [w52]
    shift-right: [w57] -> _
    shift-left: w23 -> [w48]
    shift-right: [w45] -> _
    shift-left: 0 ("queue size max") -> [w46]
    shift-right: [w40] -> _
    shift-left: w1 -> [w39]
    stop <- w59 stop-if-true
    n20 = Get Queue Status(queue=w54, error in (no error)=w52) -> (queue out=w53:refnum<queue>, error out=w51:errorcluster, # elements in queue=w43:i32)  [unwired: 1 in, 5 out]
    n21 = Not Equal To 0?(x=w43) -> (x != 0?=w49:bool)
    "Busy" <- w49
    n22 = Get Queue Status(queue=w48) -> (queue out=w47:refnum<queue>, # elements in queue=w44:i32)  [unwired: 2 in, 6 out]
    n23 = case shown="No Error" w51 {
      selector: w51 -> [w71 w76]
      tunnel: [w74 _] -> w62
      tunnel: w53 -> [w70 w78]
      tunnel: [w72 event."Shutdown - hard exit" ("task")] -> w61
      tunnel: [w73 w78] -> w60
      frame No Error {
        n24 = Dequeue Element(queue=w70, error in (no error)=w71) -> (queue out=w73:refnum<queue>, element=w72:T15, error out=w74:errorcluster)  [unwired: 1 in, 1 out]
      }
      frame Error {
        n25 = call <vilib>:"General Error Handler.vi"("error in (no error)"=w76) -> ()  [unwired: 10 in, 5 out]
        n26 = property on="Button stop" class="Bool (strict)"("Val(Sgnl)"=TRUE ("Value (Signaling)")) -> ()  [unwired: 2 in, 2 out]
      }
    }
    n27 = call "xijk_percentage_slider.vi"("queue size in"=w43, "queue size in 2"=w44, "queue size max"=w46) -> ("percentage finished"=→"Slide":dbl, "not ready?"=w41:bool, "queue size out"=w45:i32)  [unwired: 6 in]
    n28 = property on="Slide" class="Slide (strict)"("Visible"=w41) -> ()  [unwired: 2 in, 2 out]
    n29 = feedback-in #1(w49) -> ()
    n30 = feedback #1() -> (w56:bool)  [unwired: 1 in]
    n31 = Not(x=w56) -> (.not. x?=w50:bool)
    n32 = And(x=w49, y=w50) -> (x .and. y?=w55:bool)
    n33 = case shown="\"Update template\"" w61 {
      tunnel: w62 -> [w84 w109 w134 w144 w152 w166 w172 w196 w214 w324 w330 w349 w385 w389 w400 w419 w426 w465 w475 w555 w576 w617 w627 w634 w639 w652 w661 w670 w695 w726 w763 w771 w777 w788 w803 w807 w811]
      tunnel: w60 -> [_ w108 _ _ w151 _ w171 _ _ _ w329 _ _ _ w399 _ w425 _ _ _ _ w618 _ _ _ _ _ _ w694 w725 _ _ _ _ _ _ _]
      tunnel: [w87 w110 w133 w145 w153 w166 w173 w196 w206 w316 w325 w347 w385 w390 w395 w417 w421 w465 w478 w554 w577 w620 w628 w635 w639 w658 w662 w675 w693 w722 w764 w772 w777 w780 w801 w808 w812] -> w58
      tunnel: [_ _ _ _ _ TRUE _ _ _ _ _ _ _ _ _ _ _ _ _ _ _ _ _ _ _ _ _ _ _ _ _ _ _ _ _ _ _] -> w59
      tunnel: [w86 w115 w136 w143 w150 w164 w169 w195 w224 w323 w334 w358 w371 w387 w401 w414 w429 w450 w485 w560 w575 w615 w630 w632 w640 w657 w663 w678 w687 w730 w766 w774 w776 w791 w805 w810 w814] -> w57
      tunnel: w47 -> [w86 w115 w136 w143 w150 w164 w169 w195 w224 w323 w334 w358 w371 w387 w401 w414 w429 w450 w485 w560 w575 w615 w630 w632 w640 w651 w663 w678 w689 w730 w766 w774 w776 w791 w805 w810 w814]
      tunnel: w39 -> [w79 w106 w131 w142 w146 w163 w168 w194 w198 w314 w326 w353 w369 w386 w397 w412 w420 w430 w466 w551 w573 w592 w626 w631 w637 w654 w660 w665 w680 w713 w731 w770 w775 w778 w792 w809 w813]
      tunnel: [w80 w104 w131 w141 w146 w163 w167 w194 w197 w314 w331 w352 w369 w386 w397 w412 w420 w430 w466 w550 w573 w591 w626 w631 w636 w653 w660 w664 w679 w712 w731 w770 w775 w778 w792 w809 w813] -> w40
      frame "Initialise parameters" {
        n34 = Unbundle By Name(w79) -> ("GUI configuration.axes in"=w82:T8, "GUI configuration.plot colors in"=w81:T9)
        n35 = local write "axes in"(w82) -> ()
        n36 = local write "plot colors in"(w81) -> ()
        n37 = local read "Number of fluorophores"() -> (w85:u16)
        n38 = Multiply(x="Molar extinction 1", y="Quantum efficiency 1") -> (x*y=w93:sgl)
        "Brightness" <- w93
        n39 = Multiply(x="Molar extinction 2", y="Quantum efficiency 2") -> (x*y=w88:sgl)
        "Brightness 2" <- w88
        n40 = Not(x="Dual emission by cubes") -> (.not. x?=w83:bool)
        n41 = Bundle By Name(cluster=w79, "output cluster.Booleans.FRET"="FRET", "output cluster.Booleans.Dual emission by cubes"=w83, "output cluster.Booleans.Dual band filters"="Dual band filters", "output cluster.Booleans.Unknown detector"="Unknown detector", "output cluster.Integers.Light source"="Light source", "output cluster.Integers.Number of fluorophores"="Number of fluorophores", "output cluster.Integers.Wavelength of laser (nm) 1"="Wavelength of laser (nm) 1", "output cluster.Integers.Broadness of laser (nm) 1"="Broadness of laser (nm) 1", "output cluster.Integers.Wavelength of laser (nm) 2"="Wavelength of laser (nm) 2", "output cluster.Integers.Broadness of laser (nm) 2"="Broadness of laser (nm) 2", "output cluster.Doubles.Molar extinction 1"="Molar extinction 1", "output cluster.Doubles.Quantum efficiency 1"="Quantum efficiency 1", "output cluster.Doubles.Molar extinction 2"="Molar extinction 2", "output cluster.Doubles.Quantum efficiency 2"="Quantum efficiency 2") -> (w80:T1)
        n42 = call "xijk_give_warning_brightness.vi"("error in"=w84, "brightness 2 in"=w88, "Number of fluorophores"=w85, "brightness 1 in"=w93) -> ("error out"=w87:errorcluster)  [unwired: 7 in]
      }
      frame "Initialise paths" {
        n43 = Bundle By Name(cluster=w106, "output cluster 2.Excitation filter 1"="Excitation filter 1", "output cluster 2.Dichroic filter 1"="Dichroic filter 1", "output cluster 2.Emission filter 1"="Emission filter 1", "output cluster 2.Excitation filter 2"="Excitation filter 2", "output cluster 2.Dichroic filter 2"="Dichroic filter 2", "output cluster 2.Emission filter 2"="Emission filter 2", "output cluster 2.Extra em filter 1"="Extra em filter 1", "output cluster 2.Extra em filter 2"="Extra em filter 2", "output cluster 2.Detector"="Detector", "output cluster 2.Fluorophore absorption 1"="Fluorophore absorption", "output cluster 2.Fluorophore emission 1"="Fluorophore emission", "output cluster 2.Fluorophore absorption 2"="Fluorophore absorption 2", "output cluster 2.Fluorophore emission 2"="Fluorophore emission 2", "output cluster 2.Light source file"="Light source file") -> (w107:T1)
        n44 = call "xijk_combined_file_save.vi"("error in"=w109, "queue in"=w108, "Settings"=w107) -> ("error out"=w110:errorcluster, "Settings out"=w105:T1)  [unwired: 6 in, 1 out]
        n45 = local read "Path: Excitation filters"() -> (w113:path)
        n46 = local read "Path: Emission filters"() -> (w111:path)
        n47 = local read "Path: Dicroic filters"() -> (w112:path)
        n48 = local read "Path reget"() -> (w114:path)
        n49 = Bundle By Name(cluster=w105, "search parameters.Paths.Path: Excitation filters"=w113, "search parameters.Paths.Path: Dicroic filters"=w112, "search parameters.Paths.Path: Emission filters"=w111, "search parameters.Paths.Path reget"=w114) -> (w104:T1)
      }
      frame "Update filter names" {
        n50 = Unbundle By Name(w131) -> ("references"=w130:T10)
        n51 = Cluster To Array(cluster=w130) -> (array=w135:refnum<vi>[])
        n52 = for "loop over file path controls" {
          tunnel: w135 -> [w140] mode=indexing
          shift-right: [w138] -> w133
          shift-left: w134 -> [w139]
          tunnel: u32 4294967295 ("Path Text.Scroll Position") -> [w137]
          stop <- w138 stop-if-true
          n53 = property class="Path"(reference=w140, error in=w139, "Text.Scroll Position"=w137) -> (error out=w138:errorcluster)  [unwired: 1 out]
        }
      }
      frame "Get spectra from files" {
        n54 = call "xijk_get_spectra.vi"("error in"=w144, "Settings"=w142) -> ("error out"=w145:errorcluster, "Settings out"=w141:T1)  [unwired: 8 in]
      }
      frame "Shutdown" {
        n55 = Two Button Dialog(message="Do you want to save the project? ", 1:"No" ("F button name (\"Cancel\")"), 2:"Yes" ("T button name (\"OK\")")) -> (T button?=w149:bool)
        n56 = case shown="True" w149 {
          tunnel: w152 -> [w157 w160]
          tunnel: [w156 w161] -> w153
          tunnel: w151 -> [w158 w159]
          frame True {
            w155 = T15[] [enum."Save to file", enum."Shutdown - hard exit", enum."Initialise paths", enum."Get spectra from files", enum."Update filter names", enum."Calculate Xijk", enum."Create graphs"] items=["Initialise parameters", "Initialise paths", "Execute", "Hide detector", "Light source selection", "Get example list", "Set Example", "Change portrait / landscape", "Dual band cube", "Save to file", "Load from file", "Set filepaths to boxes", "1 or 2 fluorophore selection", "Update configurations", "Update template", "Calculate other values", "Update filter names", "Shutdown", "Shutdown - hard exit", "Search in filters - set parameters", "Search in filters - search", "Search in filters - get xijk", "Search in filters - reget", "Optimize - Sort table", "Get path from search", "Calculate Xijk", "Get spectra from files", "Create graphs", "Reset variables", "Tools - convert image to text", "Tools - create function", "Help - open", "Help - close", "Help - next", "Help - previous", "Help - select menu", "Export data"] ("array in")
            n57 = call "xijk_array_to_queue.vi"("error in"=w157, "array in"=w155, "queue in"=w158) -> ("error out"=w156:errorcluster)  [unwired: 7 in, 1 out]
          }
          frame False {
            n58 = Enqueue Element(queue=w159, element=event."Shutdown - hard exit", error in (no error)=w160) -> (error out=w161:errorcluster)  [unwired: 1 in, 2 out]
          }
        }
      }
      frame "Shutdown - hard exit" {
      }
      frame "Calculate Xijk" {
        n59 = Enqueue Element At Opposite End(queue=w171, element=event."Calculate other values", error in (no error)=w172) -> (error out=w173:errorcluster)  [unwired: 1 in, 2 out]
        n60 = call "xijk_calculate_effective_numbers.vi"("Settings"=w168) -> ("Effective spectral emission 2"=w174:sgl[], "Effective spectral excitation 2"=w175:sgl[], "Effective spectral emission 1"=w176:sgl[], "Effective spectral excitation 1"=w177:sgl[])  [unwired: 7 in]
        n61 = call "xijk_calc_eijk_xijk.vi"("Settings"=w168, "Effective spectral emission 2"=w174, "Effective spectral excitation 2"=w175, "Effective spectral emission 1"=w176, "Effective spectral excitation 1"=w177) -> ("Settings out"=w167:T1)  [unwired: 6 in]
        n62 = Unbundle By Name(w167) -> ("Xijk output cluster.Xijk 111"=→"Xijk 111":sgl, "Xijk output cluster.Xijk 112"=→"Xijk 112":sgl, "Xijk output cluster.Xijk 121"=→"Xijk 121":sgl, "Xijk output cluster.Xijk 122"=→"Xijk 122":sgl, "Xijk output cluster.Xijk 211"=→"Xijk 211":sgl, "Xijk output cluster.Xijk 212"=→"Xijk 212":sgl, "Xijk output cluster.Xijk 221"=→"Xijk 221":sgl, "Xijk output cluster.Xijk 222"=→"Xijk 222":sgl, "Xijk output cluster.Eijk 111"=→"Eijk 111":sgl, "Xijk output cluster.Eijk 112"=→"Eijk 112":sgl, "Xijk output cluster.Eijk 121"=→"Eijk 121":sgl, "Xijk output cluster.Eijk 122"=→"Eijk 122":sgl, "Xijk output cluster.Eijk 211"=→"Eijk 211":sgl, "Xijk output cluster.Eijk 212"=→"Eijk 212":sgl, "Xijk output cluster.Eijk 221"=→"Eijk 221":sgl, "Xijk output cluster.Eijk 222"=→"Eijk 222":sgl)
      }
      frame "Execute" {
      }
      frame "Create graphs" {
        n63 = Bundle By Name(cluster=w198, "GUI configuration.axes in"="axes in", "GUI configuration.plot colors in"="plot colors in") -> (w197:T1)
        n64 = Unbundle By Name(w197) -> ("GUI configuration.plot colors in.Line colors"=w203:u32[], "GUI configuration.plot colors in.Plot logarithmic"=w202:bool, "GUI configuration.axes in"=w201:T8)
        n65 = call "xijk_create_graphs_excitation.vi"("error in"=w214, "Settings"=w197) -> ("error out"=w227:errorcluster, "Filter cube 2 emission"=→"Filter cube 2 emission":cluster{"Y":dbl[], "Y":dbl[]}[], "Filter cube 1 emission"=→"Filter cube 1 emission":cluster{"Y":dbl[], "Y":dbl[]}[], "Filter cube 2 excitation"=→"Filter cube 2 excitation":cluster{"Y":dbl[], "Y":dbl[]}[], "Filter cube 1 excitation"=→"Filter cube 1 excitation":cluster{"Y":dbl[], "Y":dbl[]}[])  [unwired: 5 in]
        n66 = To Double Precision Float(number=w201) -> (double precision float=w219:T17)
        n67 = Select(t=0.001 ("Échelle des Y.Gamme : minimum"), s=w202, f=0.0 ("Échelle des Y.Gamme : minimum")) -> (s? t:f=w208:dbl)
        n68 = Unbundle By Name(w219) -> ("min x-axis excitation"=w223:dbl, "max x-axis excitation"=w222:dbl, "min x-axis emission"=w221:dbl, "max x-axis emission"=w220:dbl)
        n69 = Boolean To (0,1)(Boolean=w202) -> (0, 1=w226:i16)
        n70 = To Unsigned Byte Integer(number=w226) -> (unsigned 8bit integer=w225:u8)
        n71 = stacked-sequence {
          tunnel: w223 -> [w237 w244 _ _]
          tunnel: w222 -> [w236 w243 _ _]
          tunnel: w221 -> [_ _ w251 w258]
          tunnel: w220 -> [_ _ w250 w257]
          tunnel: w208 -> [w238 w245 w252 w259]
          tunnel: 1.0 ("Échelle des Y.Gamme : minimum") -> [w235 w242 w249 w256]
          tunnel: w227 -> [w234 w241 w248 w255]
          tunnel: [w233 _ _ _] -> w217
          tunnel: w225 -> [w232 w239 w246 w253]
          tunnel: [_ w240 _ _] -> w216
          tunnel: [_ _ w247 _] -> w215
          tunnel: [_ _ _ w254] -> w218
          frame #0 {
            n72 = property on="Filter cube 1 excitation" class="XYGraph (strict)"(error in=w234, "YScale.Mapping Mode"=w232, "YScale.Maximum"=w235, "YScale.Minimum"=w238, "XScale.Minimum"=w237, "XScale.Maximum"=w236) -> (error out=w233:errorcluster)  [unwired: 1 in, 1 out]
          }
          frame #1 {
            n73 = property on="Filter cube 2 excitation" class="XYGraph (strict)"(error in=w241, "YScale.Mapping Mode"=w239, "YScale.Maximum"=w242, "YScale.Minimum"=w245, "XScale.Minimum"=w244, "XScale.Maximum"=w243) -> (error out=w240:errorcluster)  [unwired: 1 in, 1 out]
          }
          frame #2 {
            n74 = property on="Filter cube 1 emission" class="XYGraph (strict)"(error in=w248, "YScale.Mapping Mode"=w246, "YScale.Maximum"=w249, "YScale.Minimum"=w252, "XScale.Minimum"=w251, "XScale.Maximum"=w250) -> (error out=w247:errorcluster)  [unwired: 1 in, 1 out]
          }
          frame #3 {
            n75 = property on="Filter cube 2 emission" class="XYGraph (strict)"(error in=w255, "YScale.Mapping Mode"=w253, "YScale.Maximum"=w256, "YScale.Minimum"=w259, "XScale.Minimum"=w258, "XScale.Maximum"=w257) -> (error out=w254:errorcluster)  [unwired: 1 in, 1 out]
          }
        }
        n76 = Build Array(w217, w216, w215, w218) -> (w204:errorcluster[])
        n77 = Merge Errors(w204) -> (w207:errorcluster)
        n78 = for {
          N: 4 -> [_]
          tunnel: "width" -> [w264] mode=indexing
          tunnel: "style" -> [w263] mode=indexing
          tunnel: w203 -> [w262]
          shift-right: [w260] -> w206
          shift-left: w207 -> [w261]
          i -> [w265]
          stop <- w260 stop-if-true
          n79 = case shown="0, Default" w265 {
            tunnel: w264 -> [w270 w282 w294 w306]
            tunnel: w263 -> [w269 w281 w293 w305]
            tunnel: w262 -> [w268 w280 w292 w304]
            tunnel: [w266 w278 w291 w302] -> w260
            tunnel: w261 -> [w267 w279 w290 w303]
            frame 0, Default {
              n80 = for {
                N: 6 -> [_]
                tunnel: w270 -> [w276] mode=indexing
                tunnel: w269 -> [w275] mode=indexing
                tunnel: w268 -> [w274] mode=indexing
                shift-right: [w272] -> w266
                shift-left: w267 -> [w273]
                i -> [w277]
                n81 = property on="Filter cube 1 excitation" class="XYGraph (strict)"(error in=w273, "Active Plot"=w277, "Plot.Plot Color"=w274, "Plot.Fill/Pt. Color"=w274, "Plot.Line Width"=w276, "Plot.Line Style"=w275) -> (error out=w272:errorcluster)  [unwired: 1 in, 1 out]
              }
            }
            frame 1 {
              n82 = for {
                N: 6 -> [_]
                tunnel: w282 -> [w284] mode=indexing
                tunnel: w281 -> [w288] mode=indexing
                tunnel: w280 -> [w287] mode=indexing
                shift-right: [w285] -> w278
                shift-left: w279 -> [w286]
                i -> [w289]
                n83 = property on="Filter cube 1 emission" class="XYGraph (strict)"(error in=w286, "Active Plot"=w289, "Plot.Plot Color"=w287, "Plot.Fill/Pt. Color"=w287, "Plot.Line Width"=w284, "Plot.Line Style"=w288) -> (error out=w285:errorcluster)  [unwired: 1 in, 1 out]
              }
            }
            frame 2 {
              n84 = for {
                N: 6 -> [_]
                tunnel: w294 -> [w300] mode=indexing
                tunnel: w293 -> [w299] mode=indexing
                tunnel: w292 -> [w298] mode=indexing
                shift-right: [w297] -> w291
                shift-left: w290 -> [w296]
                i -> [w301]
                n85 = property on="Filter cube 2 excitation" class="XYGraph (strict)"(error in=w296, "Active Plot"=w301, "Plot.Plot Color"=w298, "Plot.Fill/Pt. Color"=w298, "Plot.Line Width"=w300, "Plot.Line Style"=w299) -> (error out=w297:errorcluster)  [unwired: 1 in, 1 out]
              }
            }
            frame 3 {
              n86 = for {
                N: 6 -> [_]
                tunnel: w306 -> [w312] mode=indexing
                tunnel: w305 -> [w311] mode=indexing
                tunnel: w304 -> [w310] mode=indexing
                shift-right: [w308] -> w302
                shift-left: w303 -> [w309]
                i -> [w313]
                n87 = property on="Filter cube 2 emission" class="XYGraph (strict)"(error in=w309, "Active Plot"=w313, "Plot.Plot Color"=w310, "Plot.Fill/Pt. Color"=w310, "Plot.Line Width"=w312, "Plot.Line Style"=w311) -> (error out=w308:errorcluster)  [unwired: 1 in, 1 out]
              }
            }
          }
        }
      }
      frame "1 or 2 fluorophore selection" {
        w318 = u16 2 ("y")
        n88 = local read "Number of fluorophores"() -> (w320:u16)
        n89 = Equal To 0?(x=w320) -> (x = 0?=w322:bool)
        n90 = property on="fluorophores hide box" class="Bool"(error in=w324, "Visible"=w322) -> (error out=w321:errorcluster)  [unwired: 1 in, 1 out]
        n91 = Multiply(x=w320, y=w318) -> (x*y=w319:u16)
        n92 = Subtract(x=w318, y=w319) -> (x-y=w315:u16)
        n93 = property on="Filter cube 2 excitation" class="XYGraph (strict)"(error in=w321, "DisabledEnum"=w315) -> (error out=w317:errorcluster)  [unwired: 1 in, 1 out]
        n94 = property on="Filter cube 2 emission" class="XYGraph (strict)"(error in=w317, "DisabledEnum"=w315) -> (error out=w316:errorcluster)  [unwired: 1 in, 1 out]
      }
      frame "Update configurations" {
        w328 = T15[] [enum."Initialise parameters", enum."Initialise paths", enum."Light source selection", enum."Update filter names", enum."Get spectra from files", enum."Calculate Xijk", enum."Create graphs"] items=["Initialise parameters", "Initialise paths", "Execute", "Hide detector", "Light source selection", "Get example list", "Set Example", "Change portrait / landscape", "Dual band cube", "Save to file", "Load from file", "Set filepaths to boxes", "1 or 2 fluorophore selection", "Update configurations", "Update template", "Calculate other values", "Update filter names", "Shutdown", "Shutdown - hard exit", "Search in filters - set parameters", "Search in filters - search", "Search in filters - get xijk", "Search in filters - reget", "Optimize - Sort table", "Get path from search", "Calculate Xijk", "Get spectra from files", "Create graphs", "Reset variables", "Tools - convert image to text", "Tools - create function", "Help - open", "Help - close", "Help - next", "Help - previous", "Help - select menu", "Export data"]
        n95 = call "xijk_array_to_queue.vi"("error in"=w330, "array in"=w328, "queue in"=w329) -> ("error out"=w325:errorcluster)  [unwired: 7 in, 1 out]
        n96 = Unbundle By Name(w326) -> ("GUI configuration.axes in.precision of results"=w332:u8)
        n97 = local read "Select template"() -> (w327:u16)
        n98 = call "xijk_hide_template_boxes.vi"("number"=w332, "template selector in"=w327) -> ("table for calculation automagic out"=w333:i32[], "enable array out"=w343:T18, "concatenated string"=w344:string)  [unwired: 6 in, 1 out]
        n99 = Index Array(array=w343) -> (element #1=w335:T19, element #2=w336:T19, element #3=w337:T19, element #4=w338:T19, element #5=w339:T19, element #6=w340:T19, element #7=w341:T19, element #8=w342:T19)  [unwired: 8 in]
        n100 = property on="Xijk 111" class="DigNum (strict)"("Disabled"=w335, "FormatString"=w344) -> ()  [unwired: 2 in, 2 out]
        n101 = property on="Xijk 112" class="DigNum (strict)"("Disabled"=w336, "FormatString"=w344) -> ()  [unwired: 2 in, 2 out]
        n102 = property on="Xijk 121" class="DigNum (strict)"("Disabled"=w337, "FormatString"=w344) -> ()  [unwired: 2 in, 2 out]
        n103 = property on="Xijk 122" class="DigNum (strict)"("Disabled"=w338, "FormatString"=w344) -> ()  [unwired: 2 in, 2 out]
        n104 = property on="Xijk 212" class="DigNum (strict)"("Disabled"=w339, "FormatString"=w344) -> ()  [unwired: 2 in, 2 out]
        n105 = property on="Xijk 211" class="DigNum (strict)"("Disabled"=w340, "FormatString"=w344) -> ()  [unwired: 2 in, 2 out]
        n106 = property on="Xijk 222" class="DigNum (strict)"("Disabled"=w341, "FormatString"=w344) -> ()  [unwired: 2 in, 2 out]
        n107 = property on="Xijk 221" class="DigNum (strict)"("Disabled"=w342, "FormatString"=w344) -> ()  [unwired: 2 in, 2 out]
        n108 = Bundle By Name(cluster=w326, "search parameters.table for calculation automagic"=w333) -> (w331:T1)
        n109 = property on="Eijk 111" class="DigNum (strict)"("Disabled"=w335, "FormatString"=w344) -> ()  [unwired: 2 in, 2 out]
        n110 = property on="Eijk 112" class="DigNum (strict)"("Disabled"=w336, "FormatString"=w344) -> ()  [unwired: 2 in, 2 out]
        n111 = property on="Eijk 121" class="DigNum (strict)"("Disabled"=w337, "FormatString"=w344) -> ()  [unwired: 2 in, 2 out]
        n112 = property on="Eijk 122" class="DigNum (strict)"("Disabled"=w338, "FormatString"=w344) -> ()  [unwired: 2 in, 2 out]
        n113 = property on="Eijk 212" class="DigNum (strict)"("Disabled"=w339, "FormatString"=w344) -> ()  [unwired: 2 in, 2 out]
        n114 = property on="Eijk 211" class="DigNum (strict)"("Disabled"=w340, "FormatString"=w344) -> ()  [unwired: 2 in, 2 out]
        n115 = property on="Eijk 222" class="DigNum (strict)"("Disabled"=w341, "FormatString"=w344) -> ()  [unwired: 2 in, 2 out]
        n116 = property on="Eijk 221" class="DigNum (strict)"("Disabled"=w342, "FormatString"=w344) -> ()  [unwired: 2 in, 2 out]
      }
      frame "Update template" {
        n117 = Unbundle By Name(w353) -> ("GUI configuration.axes in.precision of results"=w354:u8)
        n118 = call "xijk_template_select_booleans.vi"("Select template"="Select template") -> ("FRET?"=w356:bool, "Dual emission?"=w346:bool, "Number of fluorophores out"=w348:i32, "Light source out"=w355:i32)  [unwired: 7 in]
        n119 = property on="Light source" class="Ring (strict)"(error in=w349, "Value"=w355) -> (error out=w347:errorcluster)  [unwired: 1 in, 1 out]
        n120 = Not(x=w346) -> (.not. x?=w345:bool)
        n121 = Bundle By Name(cluster=w353, "output cluster.Integers.Template"="Select template") -> (w351:T1)
        n122 = local write "Number of fluorophores"(w348) -> ()
        n123 = local write "Dual emission by cubes"(w345) -> ()
        n124 = local write "FRET"(w356) -> ()
        n125 = call "xijk_hide_template_boxes.vi"("number"=w354, "template selector in"="Select template") -> ("table for calculation automagic out"=w357:i32[], "enable array out"=w367:T18, "concatenated string"=w368:string)  [unwired: 6 in, 1 out]
        n126 = Index Array(array=w367) -> (element #1=w359:T19, element #2=w360:T19, element #3=w361:T19, element #4=w362:T19, element #5=w363:T19, element #6=w364:T19, element #7=w365:T19, element #8=w366:T19)  [unwired: 8 in]
        n127 = property on="Xijk 111" class="DigNum (strict)"("Disabled"=w359, "FormatString"=w368) -> ()  [unwired: 2 in, 2 out]
        n128 = property on="Xijk 112" class="DigNum (strict)"("Disabled"=w360, "FormatString"=w368) -> ()  [unwired: 2 in, 2 out]
        n129 = property on="Xijk 121" class="DigNum (strict)"("Disabled"=w361, "FormatString"=w368) -> ()  [unwired: 2 in, 2 out]
        n130 = property on="Xijk 122" class="DigNum (strict)"("Disabled"=w362, "FormatString"=w368) -> ()  [unwired: 2 in, 2 out]
        n131 = property on="Xijk 212" class="DigNum (strict)"("Disabled"=w363, "FormatString"=w368) -> ()  [unwired: 2 in, 2 out]
        n132 = property on="Xijk 211" class="DigNum (strict)"("Disabled"=w364, "FormatString"=w368) -> ()  [unwired: 2 in, 2 out]
        n133 = property on="Xijk 222" class="DigNum (strict)"("Disabled"=w365, "FormatString"=w368) -> ()  [unwired: 2 in, 2 out]
        n134 = property on="Xijk 221" class="DigNum (strict)"("Disabled"=w366, "FormatString"=w368) -> ()  [unwired: 2 in, 2 out]
        n135 = Bundle By Name(cluster=w351, "search parameters.table for calculation automagic"=w357) -> (w352:T1)
        n136 = property on="Eijk 111" class="DigNum (strict)"("Disabled"=w359, "FormatString"=w368) -> ()  [unwired: 2 in, 2 out]
        n137 = property on="Eijk 112" class="DigNum (strict)"("Disabled"=w360, "FormatString"=w368) -> ()  [unwired: 2 in, 2 out]
        n138 = property on="Eijk 121" class="DigNum (strict)"("Disabled"=w361, "FormatString"=w368) -> ()  [unwired: 2 in, 2 out]
        n139 = property on="Eijk 122" class="DigNum (strict)"("Disabled"=w362, "FormatString"=w368) -> ()  [unwired: 2 in, 2 out]
        n140 = property on="Eijk 212" class="DigNum (strict)"("Disabled"=w363, "FormatString"=w368) -> ()  [unwired: 2 in, 2 out]
        n141 = property on="Eijk 211" class="DigNum (strict)"("Disabled"=w364, "FormatString"=w368) -> ()  [unwired: 2 in, 2 out]
        n142 = property on="Eijk 222" class="DigNum (strict)"("Disabled"=w365, "FormatString"=w368) -> ()  [unwired: 2 in, 2 out]
        n143 = property on="Eijk 221" class="DigNum (strict)"("Disabled"=w366, "FormatString"=w368) -> ()  [unwired: 2 in, 2 out]
        "Result template" <- "Select template"
      }
      frame "Calculate other values" {
        n144 = call "xijk_calculate_effective_numbers.vi"("Settings"=w369) -> ("Effective spectral emission 2"=w381:sgl[], "Effective spectral excitation 2"=w382:sgl[], "Effective spectral emission 1"=w383:sgl[], "Effective spectral excitation 1"=w384:sgl[])  [unwired: 7 in]
        n145 = call "xijk_calc_other_parameters.vi"("Settings"=w369, "Effective spectral emission 2"=w381, "Effective spectral excitation 2"=w382, "Effective spectral emission 1"=w383, "Effective spectral excitation 1"=w384) -> ("array out"=w380:dbl[])  [unwired: 6 in]
        n146 = Index Array(array=w380) -> (element #1=→"excitation light bleed through":dbl, element #2=→"% Absorption":dbl, element #3=→"% Emission":dbl, element #4=→"% Absorption":dbl, element #5=→"% Emission":dbl, element #6=→"excitation light bleed through 2":dbl, element #7=→"Spectral overlap efficiency":dbl, element #8=→"% Green emission in red channel":dbl, element #9=→"% Red emission in green channel":dbl)  [unwired: 9 in]
      }
      frame "Hide detector" {
        n147 = local read "hide detector box?"() -> (w388:bool)
        n148 = property on="detector hide box" class="Bool"(error in=w389, "Visible"=w388) -> (error out=w390:errorcluster)  [unwired: 1 in, 1 out]
      }
      frame "Light source selection" {
        n149 = Enqueue Element At Opposite End(queue=w399, element=event."Initialise parameters", error in (no error)=w400) -> (error out=w393:errorcluster)  [unwired: 1 in, 2 out]
        n150 = property on="Light source" class="Ring (strict)"(error in=w393) -> (error out=w392:errorcluster, "Value"=w394:u16)  [unwired: 1 in, 1 out]
        n151 = case "Which case?" shown="1" w394 {
          tunnel: [enum32{"Page 1", "Page 2"}."Page 1" ("Tab Control") enum32{"Page 1", "Page 2"}."Page 2" ("Tab Control") enum32{"Page 1", "Page 2"}."Page 2" ("Tab Control")] -> w396
          tunnel: [TRUE ("Visible") TRUE ("Visible") FALSE ("Visible")] -> w402
          tunnel: w392 -> [w403 w406 w409]
          tunnel: [w403 w406 w409] -> w391
          frame 0, Default {
          }
          frame 1 {
          }
          frame 2 {
          }
        }
        "Tab Control" <- w396
        n152 = property on="laser hide box" class="Bool"(error in=w391, "Visible"=w402) -> (error out=w395:errorcluster)  [unwired: 1 in, 1 out]
      }
      frame "Get example list" {
        n153 = Current VI's Path() -> (path=w413:path)
        n154 = call "xijk_create_example_list.vi"("error in"=w419, "path"=w413) -> ("error out"=w418:errorcluster, "example list array out"=w415:string[], "filepath array out"=→"Table of settings":path[])  [unwired: 7 in]
        n155 = property on="Examples" class="Ring (strict)"(error in=w418, "Strings []"=w415) -> (error out=w417:errorcluster)  [unwired: 1 in, 1 out]
      }
      frame "Set Example" {
        n156 = Enqueue Element(queue=w425, element=event."Load from file", error in (no error)=w426) -> (error out=w423:errorcluster)  [unwired: 1 in, 2 out]
        n157 = local read "Table of settings"() -> (w428:path[])
        n158 = call "xijk_get_example_load_file.vi"("error in"=w423, "Examples"="Examples", "Table of settings"=w428) -> ("error out"=w421:errorcluster, "appended path"=w427:path)  [unwired: 7 in]
        n159 = local write "start path"(w427) -> ()
      }
      frame "Set filepaths to boxes" {
        n160 = Unbundle By Name(w430) -> ("search parameters.Paths.Path: Excitation filters"=w449:path, "search parameters.Paths.Path: Dicroic filters"=w448:path, "search parameters.Paths.Path: Emission filters"=w447:path, "search parameters.Paths.Path reget"=w446:path, "search parameters.Integers.Select result number"=w445:u32, "search parameters.boolean selector array"=w444:bool[])
        n161 = Index Array(array=w444) -> (element #1=w443:bool, element #2=w442:bool, element #3=w441:bool, element #4=w440:bool, element #5=w439:bool, element #6=w438:bool)  [unwired: 6 in]
        n162 = local write "Select result number"(w445) -> ()
        n163 = local write "Path: Excitation filters"(w449) -> ()
        n164 = local write "Path: Dicroic filters"(w448) -> ()
        n165 = local write "Path: Emission filters"(w447) -> ()
        n166 = local write "Path reget"(w446) -> ()
        n167 = local write "1. Excitation"(w443) -> ()
        n168 = local write "1. Dichroic"(w442) -> ()
        n169 = local write "1. Emission"(w441) -> ()
        n170 = local write "2. Excitation"(w440) -> ()
        n171 = local write "2. Dichroic"(w439) -> ()
        n172 = local write "2. Emission"(w438) -> ()
        n173 = Unbundle By Name(w430) -> ("output cluster.Integers.Light source"=w437:u16, "output cluster.Integers.Number of fluorophores"=w436:u16, "output cluster.Integers.Wavelength of laser (nm) 1"=w435:u16, "output cluster.Integers.Broadness of laser (nm) 1"=w434:sgl, "output cluster.Integers.Wavelength of laser (nm) 2"=w433:u16, "output cluster.Integers.Broadness of laser (nm) 2"=w432:sgl, "output cluster.Integers.Template"=w431:u16)
        n174 = Unbundle By Name(w430) -> ("output cluster 2.Excitation filter 1"=w464:path, "output cluster 2.Dichroic filter 1"=w463:path, "output cluster 2.Emission filter 1"=w462:path, "output cluster 2.Excitation filter 2"=w461:path, "output cluster 2.Dichroic filter 2"=w460:path, "output cluster 2.Emission filter 2"=w459:path, "output cluster 2.Extra em filter 1"=w458:path, "output cluster 2.Extra em filter 2"=w457:path, "output cluster 2.Fluorophore absorption 1"=w456:path, "output cluster 2.Fluorophore emission 1"=w455:path, "output cluster 2.Fluorophore absorption 2"=w454:path, "output cluster 2.Fluorophore emission 2"=w453:path, "output cluster 2.Detector"=w452:path, "output cluster 2.Light source file"=w451:path)
        n175 = local write "Light source"(w437) -> ()
        n176 = local write "Number of fluorophores"(w436) -> ()
        n177 = local write "Wavelength of laser (nm) 1"(w435) -> ()
        n178 = local write "Broadness of laser (nm) 1"(w434) -> ()
        n179 = local write "Wavelength of laser (nm) 2"(w433) -> ()
        n180 = local write "Broadness of laser (nm) 2"(w432) -> ()
        n181 = local write "Select template"(w431) -> ()
        n182 = local write "Excitation filter 1"(w464) -> ()
        n183 = local write "Dichroic filter 1"(w463) -> ()
        n184 = local write "Emission filter 1"(w462) -> ()
        n185 = local write "Excitation filter 2"(w461) -> ()
        n186 = local write "Dichroic filter 2"(w460) -> ()
        n187 = local write "Emission filter 2"(w459) -> ()
        n188 = local write "Extra em filter 1"(w458) -> ()
        n189 = local write "Extra em filter 2"(w457) -> ()
        n190 = local write "Fluorophore absorption"(w456) -> ()
        n191 = local write "Fluorophore emission"(w455) -> ()
        n192 = local write "Fluorophore absorption 2"(w454) -> ()
        n193 = local write "Fluorophore emission 2"(w453) -> ()
        n194 = local write "Detector"(w452) -> ()
        n195 = local write "Light source file"(w451) -> ()
      }
      frame "Change portrait / landscape" {
        w479 = 463 ("y2")
        w480 = 702 ("x 3")
        w482 = 199 ("y2")
        w481 = 402 ("x 2")
        n196 = property class="VI"(error in=w475) -> (error out=w471:errorcluster, "Front Panel.PanelBounds"=w472:T20)  [unwired: 1 in, 1 out]
        n197 = local read "plot colors in"() -> (w483:T9)
        n198 = Unbundle By Name(w483) -> ("Lanscape Portrait"=w484:bool)
        n199 = Unbundle By Name(w472) -> ("left"=w474:i16, "top"=w473:i16)
        n200 = case "Portrait?" shown="True" w484 {
          tunnel: w481 -> [w522 w549]
          tunnel: w482 -> [w520 w547]
          tunnel: 306 ("x") -> [w506 w533]
          tunnel: [w521 w548] -> w494
          tunnel: [w519 w546] -> w493
          tunnel: 269 ("y") -> [w505 w532]
          tunnel: w480 -> [w517 w545]
          tunnel: w482 -> [w511 w544]
          tunnel: [w518 w543] -> w491
          tunnel: [w512 w542] -> w490
          tunnel: w481 -> [w516 w541]
          tunnel: [w515 w540] -> w489
          tunnel: w479 -> [w514 w539]
          tunnel: [w513 w538] -> w488
          tunnel: w480 -> [w510 w537]
          tunnel: [w509 w536] -> w487
          tunnel: w479 -> [w508 w535]
          tunnel: [w507 w534] -> w486
          tunnel: [w496 w523] -> w476
          tunnel: [T16 {"Horizontal"=84, "Vertical"=-10} ("Origin") T16 {"Horizontal"=84, "Vertical"=-81} ("Origin")] -> w477
          tunnel: w474 -> [w503 w530]
          tunnel: w473 -> [w501 w528]
          tunnel: w472 -> [w499 w526]
          frame True {
            n201 = Add(x=w501, y=i16 1015) -> (x+y=w497:i16)
            n202 = Add(x=w503, y=i16 624) -> (x+y=w498:i16)
            n203 = Bundle By Name(cluster=w499, "right"=w498, "bottom"=w497) -> (w496:T20)
            n204 = Subtract(x=w522, y=w506) -> (x-y=w521:i32)
            n205 = Add(x=w520, y=w505) -> (x+y=w519:i32)
            n206 = Subtract(x=w517, y=w506) -> (x-y=w518:i32)
            n207 = Add(x=w511, y=w505) -> (x+y=w512:i32)
            n208 = Subtract(x=w516, y=w506) -> (x-y=w515:i32)
            n209 = Add(x=w514, y=w505) -> (x+y=w513:i32)
            n210 = Subtract(x=w510, y=w506) -> (x-y=w509:i32)
            n211 = Add(x=w508, y=w505) -> (x+y=w507:i32)
          }
          frame False {
            n212 = Add(x=w530, y=i16 1235) -> (x+y=w525:i16)
            n213 = Add(x=w528, y=i16 548) -> (x+y=w524:i16)
            n214 = Bundle By Name(cluster=w526, "right"=w525, "bottom"=w524) -> (w523:T20)
            n215 = Add(x=w549, y=w533) -> (x+y=w548:i32)
            n216 = Subtract(x=w547, y=w532) -> (x-y=w546:i32)
            n217 = Add(x=w545, y=w533) -> (x+y=w543:i32)
            n218 = Subtract(x=w544, y=w532) -> (x-y=w542:i32)
            n219 = Add(x=w541, y=w533) -> (x+y=w540:i32)
            n220 = Subtract(x=w539, y=w532) -> (x-y=w538:i32)
            n221 = Add(x=w537, y=w533) -> (x+y=w536:i32)
            n222 = Subtract(x=w535, y=w532) -> (x-y=w534:i32)
          }
        }
        n223 = property on="Filter cube 1 excitation" class="XYGraph (strict)"("Left"=w494, "Top"=w493) -> (error out=w469:errorcluster)  [unwired: 2 in, 1 out]
        n224 = property on="Filter cube 2 excitation" class="XYGraph (strict)"(error in=w469, "Left"=w491, "Top"=w490) -> (error out=w468:errorcluster)  [unwired: 1 in, 1 out]
        n225 = property on="Filter cube 1 emission" class="XYGraph (strict)"(error in=w468, "Left"=w489, "Top"=w488) -> (error out=w467:errorcluster)  [unwired: 1 in, 1 out]
        n226 = property on="Filter cube 2 emission" class="XYGraph (strict)"(error in=w467, "Left"=w487, "Top"=w486) -> ()  [unwired: 1 in, 2 out]
        n227 = property on="Pane" class="Pane"(error in=w471, "Origin"=w477) -> (error out=w470:errorcluster)  [unwired: 1 in, 1 out]
        n228 = property class="VI"(error in=w470, "Front Panel.PanelBounds"=w476) -> (error out=w478:errorcluster)  [unwired: 1 in, 1 out]
      }
      frame "Dual band cube" {
        n229 = local read "Dual band filters"() -> (w552:bool)
        n230 = Boolean To (0,1)(Boolean=w552) -> (0, 1=w559:i16)
        n231 = case shown="True" w552 {
          tunnel: w551 -> [w561 w566]
          tunnel: [w561 w565] -> w550
          frame False {
          }
          frame True {
            n232 = Unbundle By Name(w566) -> ("output cluster 2.Excitation filter 1"=w564:path, "output cluster 2.Dichroic filter 1"=w563:path, "output cluster 2.Emission filter 1"=w562:path)
            n233 = Bundle By Name(cluster=w566, "output cluster 2.Excitation filter 2"=w564, "output cluster 2.Dichroic filter 2"=w563, "output cluster 2.Emission filter 2"=w562) -> (w565:T1)
          }
        }
        n234 = Multiply(x=w559, y=i16 2) -> (x*y=w553:i16)
        n235 = property on="Excitation filter 2" class="Path"(error in=w555, "DisabledEnum"=w553) -> (error out=w557:errorcluster)  [unwired: 1 in, 1 out]
        n236 = property on="Dichroic filter 2" class="Path"(error in=w557, "DisabledEnum"=w553) -> (error out=w556:errorcluster)  [unwired: 1 in, 1 out]
        n237 = property on="Emission filter 2" class="Path"(error in=w556, "DisabledEnum"=w553) -> (error out=w554:errorcluster)  [unwired: 1 in, 1 out]
      }
      frame "Save to file" {
        n238 = Unbundle By Name(w573) -> ("GUI configuration"=w570:T7, "search parameters"=w569:T2, "output cluster"=w567:T3, "output cluster 2"=w568:T4)
        n239 = local read "Project name"() -> (w571:string)
        n240 = Bundle(cluster="save cluster", "Project name"=w571, "configuration"=w570, "search paths in"=w569, "spectra parameters in"=w567, "filepaths in"=w568) -> (w574:T11)
        n241 = call "xijk_save_to_file.vi"("error in"=w576, "save cluster"=w574) -> ("error out"=w577:errorcluster)  [unwired: 9 in]
      }
      frame "Load from file" {
        w616 = T15[] [enum."Set filepaths to boxes", enum."Initialise parameters", enum."Initialise paths", enum."Get spectra from files", enum."Update filter names", enum."Calculate Xijk", enum."Update configurations", enum."Light source selection", enum."1 or 2 fluorophore selection", enum."Create graphs"] items=["Initialise parameters", "Initialise paths", "Execute", "Hide detector", "Light source selection", "Get example list", "Set Example", "Change portrait / landscape", "Dual band cube", "Save to file", "Load from file", "Set filepaths to boxes", "1 or 2 fluorophore selection", "Update configurations", "Update template", "Calculate other values", "Update filter names", "Shutdown", "Shutdown - hard exit", "Search in filters - set parameters", "Search in filters - search", "Search in filters - get xijk", "Search in filters - reget", "Optimize - Sort table", "Get path from search", "Calculate Xijk", "Get spectra from files", "Create graphs", "Reset variables", "Tools - convert image to text", "Tools - create function", "Help - open", "Help - close", "Help - next", "Help - previous", "Help - select menu", "Export data"]
        n242 = Unbundle By Name(w592) -> ("GUI configuration"=w587:T7, "search parameters"=w588:T2, "output cluster"=w589:T3, "output cluster 2"=w590:T4)
        n243 = local read "Project name"() -> (w586:string)
        n244 = call "xijk_array_to_queue.vi"("error in"=w617, "array in"=w616, "queue in"=w618) -> ("error out"=w619:errorcluster)  [unwired: 7 in, 1 out]
        n245 = local read "save cluster"() -> (w578:T11)
        n246 = Bundle(cluster=w578, "Project name"=w586, "configuration"=w587, "search paths in"=w588, "spectra parameters in"=w589, "filepaths in"=w590) -> (w597:T11)
        n247 = call "xijk_load_from_file_choose_file.vi"("error in"=w619, "start path"="start path", "save cluster in"=w597) -> ("error out"=w620:errorcluster, "path out"=w612:path, "save cluster out"=w614:T11)  [unwired: 6 in]
        n248 = Unbundle(w614) -> ("Project name"=w581:string, "configuration"=w582:T7, "search paths in"=w583:T2, "spectra parameters in"=w584:T3, "filepaths in"=w585:T4)
        n249 = local write "Project name"(w581) -> ()
        n250 = local write "start path"(w612) -> ()
        n251 = To Variant(anything=w582) -> (Variant=w596:variant)
        n252 = Bundle By Name(cluster=w592, "GUI configuration"=w582, "search parameters"=w583, "output cluster"=w584, "output cluster 2"=w585) -> (w591:T1)
        n253 = Variant To Flattened String(Variant=w596) -> (data string=w594:string)  [unwired: 1 out]
        n254 = Unbundle By Name(w584) -> ("Booleans.Unknown detector"=w610:bool, "Booleans.Dual band filters"=w609:bool, "Booleans.Dual emission by cubes"=w580:bool, "Booleans.FRET"=w611:bool, "Integers.Light source"=w608:u16, "Integers.Number of fluorophores"=w607:u16, "Integers.Wavelength of laser (nm) 1"=w606:u16, "Integers.Broadness of laser (nm) 1"=w605:sgl, "Integers.Wavelength of laser (nm) 2"=w604:u16, "Integers.Broadness of laser (nm) 2"=w603:sgl, "Integers.Template"=w598:u16, "Doubles.Molar extinction 1"=w602:sgl, "Doubles.Molar extinction 2"=w601:sgl, "Doubles.Quantum efficiency 1"=w600:sgl, "Doubles.Quantum efficiency 2"=w599:sgl)
        n255 = Equal?(x="\u0000\u0000\u0000\u0000\u0000\u0000\u0000\u0000\u0000\u0000\u0000\u0000\u0000\u0000\u0000\u0000" ("String"), y=w594) -> (x = y?=w593:bool)
        n256 = case shown="True" w593 {
          tunnel: w582 -> [w623 _]
          frame False {
            n257 = Unbundle By Name(w623) -> ("axes in"=w622:T8, "plot colors in"=w621:T9)
            n258 = local write "axes in"(w622) -> ()
            n259 = local write "plot colors in"(w621) -> ()
          }
          frame True {
            n260 = invoke on="axes in" class="Clust (strict)" method="Reinit To Default"() -> (error out=w624:errorcluster)  [unwired: 3 in, 2 out]
            n261 = invoke on="Line colors" class="Arr (strict)" method="Reinit To Default"(error in=w624) -> ()  [unwired: 2 in, 3 out]
          }
        }
        n262 = Not(x=w580) -> (.not. x?=w579:bool)
        n263 = local write "Unknown detector"(w610) -> ()
        n264 = local write "Dual band filters"(w609) -> ()
        n265 = local write "Dual emission by cubes"(w579) -> ()
        n266 = local write "FRET"(w611) -> ()
        n267 = local write "Light source"(w608) -> ()
        n268 = local write "Number of fluorophores"(w607) -> ()
        n269 = local write "Wavelength of laser (nm) 1"(w606) -> ()
        n270 = local write "Broadness of laser (nm) 1"(w605) -> ()
        n271 = local write "Wavelength of laser (nm) 2"(w604) -> ()
        n272 = local write "Broadness of laser (nm) 2"(w603) -> ()
        n273 = local write "Result template"(w598) -> ()
        n274 = local write "Select template"(w598) -> ()
        n275 = local write "Molar extinction 1"(w602) -> ()
        n276 = local write "Molar extinction 2"(w601) -> ()
        n277 = local write "Quantum efficiency 1"(w600) -> ()
        n278 = local write "Quantum efficiency 2"(w599) -> ()
      }
      frame "Export data" {
        n279 = Unbundle By Name(w626) -> ("Xijk output cluster"=w625:T6)
        n280 = Flatten To XML(anything=w625) -> (xml string=w629:string)
        n281 = call-poly <vilib>:"Write to XML File.vi"("error in (no error)"=w627, "XML Input"=w629) -> ("error out"=w628:errorcluster)  [unwired: 7 in, 2 out]
      }
      frame "Reset variables" {
        w633 = u8 0 items=["none", "CFP", "CFP-YFP", "FITC-TxRed", "YFP"] ("Examples")
        n282 = property on="Examples" class="Ring (strict)"(error in=w634, "Val(Sgnl)"=w633) -> (error out=w635:errorcluster)  [unwired: 1 in, 1 out]
      }
      frame "Search in filters - set parameters" {
        n283 = Build Array("1. Excitation", "1. Dichroic", "1. Emission", "2. Excitation", "2. Dichroic", "2. Emission") -> (w641:bool[])
        n284 = Bundle By Name(cluster=w637, "search parameters.boolean selector array"=w641, "search parameters.Paths.Path: Excitation filters"="Path: Excitation filters", "search parameters.Paths.Path: Dicroic filters"="Path: Dicroic filters", "search parameters.Paths.Path: Emission filters"="Path: Emission filters", "search parameters.Integers.Select result number"="Select result number") -> (w636:T1)
      }
      frame "Search in filters - search" {
        n285 = call "xijk_automatic_read_3_tables.vi"("error in"=w652, "Settings"=w654) -> ("error out"=w659:errorcluster, "correct paths?"=w656:bool, "Settings out"=w655:T1)  [unwired: 7 in]
        n286 = call "xijk_create_search_list.vi"("error in"=w659, "correct paths?"=w656, "queue in"=w651, "Settings"=w655) -> ("error out"=w658:errorcluster, "queue out"=w657:refnum<queue>, "Settings out"=w653:T1)  [unwired: 5 in]
      }
      frame "Search in filters - get xijk" {
        n287 = call "xijk_save_search_xijk_to_file.vi"("error in"=w661, "Settings"=w660) -> ("error out"=w662:errorcluster)  [unwired: 9 in]
      }
      frame "Search in filters - reget" {
        n288 = local read "Select result number"() -> (w666:u32)
        n289 = Bundle By Name(cluster=w665, "search parameters.Integers.Select result number"=w666) -> (w667:T1)
        n290 = local read "Select template"() -> (w677:u16)
        n291 = call "xijk_get_search_table.vi"("template in"=w677, "error in"=w670, "Settings"=w667) -> ("error out"=w671:errorcluster, "Settings out"=w669:T1)  [unwired: 7 in]
        n292 = Unbundle By Name(w669) -> ("search parameters.Paths.Path reget"=w672:path, "search parameters.table for calculation automagic"=w673:i32[])
        n293 = call "xijk_select_best_filter.vi"("error in"=w671, "calculation table"=w673, "Column Sort Order"=i32[] [22], "file to be analyzed"=w672) -> ("error out"=w676:errorcluster, "sorted output paths table"=w674:string[][])  [unwired: 6 in]
        n294 = call "xijk_search_sorttable_to_paths.vi"("error in"=w676, "sorted output paths table"=w674, "Settings"=w669) -> ("error out"=w675:errorcluster, "Settings out"=w664:T1)  [unwired: 7 in]
      }
      frame "Get path from search" {
        w696 = T15[] [enum."Set filepaths to boxes", enum."Initialise paths", enum."Get spectra from files", enum."Update filter names", enum."Calculate Xijk", enum."Search in filters - get xijk"] items=["Initialise parameters", "Initialise paths", "Execute", "Hide detector", "Light source selection", "Get example list", "Set Example", "Change portrait / landscape", "Dual band cube", "Save to file", "Load from file", "Set filepaths to boxes", "1 or 2 fluorophore selection", "Update configurations", "Update template", "Calculate other values", "Update filter names", "Shutdown", "Shutdown - hard exit", "Search in filters - set parameters", "Search in filters - search", "Search in filters - get xijk", "Search in filters - reget", "Optimize - Sort table", "Get path from search", "Calculate Xijk", "Get spectra from files", "Create graphs", "Reset variables", "Tools - convert image to text", "Tools - create function", "Help - open", "Help - close", "Help - next", "Help - previous", "Help - select menu", "Export data"]
        n295 = call "xijk_array_to_queue.vi"("error in"=w695, "array in"=w696, "queue in"=w694) -> ("error out"=w686:errorcluster, "queue out"=w684:refnum<queue>)  [unwired: 7 in]
        n296 = case shown="True" "fast search?" {
          tunnel: w686 -> [w701 w702]
          tunnel: [w700 w702] -> w685
          tunnel: w684 -> [w699 w703]
          tunnel: [w698 w703] -> w683
          frame False {
            n297 = Enqueue Element(queue=w699, element=event."Create graphs", error in (no error)=w701) -> (queue out=w698:refnum<queue>, error out=w700:errorcluster)  [unwired: 1 in, 1 out]
          }
          frame True {
          }
        }
        n298 = Dequeue Element(queue=w689, error in (no error)=w685) -> (queue out=w688:refnum<queue>, element=w681:T4, error out=w692:errorcluster)  [unwired: 1 in, 1 out]
        n299 = Bundle By Name(cluster=w680, "output cluster 2"=w681) -> (w679:T1)
        n300 = Get Queue Status(queue=w688, error in (no error)=w692) -> (queue out=w687:refnum<queue>, error out=w691:errorcluster, # elements in queue=w690:i32)  [unwired: 1 in, 5 out]
        n301 = case "Loop while queue is not empty" shown="Default" w690 {
          tunnel: w691 -> [w707 w711]
          tunnel: [w706 w710] -> w693
          tunnel: w683 -> [w705 w709]
          frame Default {
            n302 = Enqueue Element(queue=w705, element=event."Get path from search", error in (no error)=w707) -> (error out=w706:errorcluster)  [unwired: 1 in, 2 out]
          }
          frame 0 {
            n303 = Enqueue Element(queue=w709, element=event."Optimize - Sort table", error in (no error)=w711) -> (error out=w710:errorcluster)  [unwired: 1 in, 2 out]
          }
        }
      }
      frame "Optimize - Sort table" {
        w724 = T15[] [enum."Set filepaths to boxes", enum."Initialise parameters", enum."Initialise paths", enum."Get spectra from files", enum."Update filter names", enum."Calculate Xijk", enum."Create graphs"] items=["Initialise parameters", "Initialise paths", "Execute", "Hide detector", "Light source selection", "Get example list", "Set Example", "Change portrait / landscape", "Dual band cube", "Save to file", "Load from file", "Set filepaths to boxes", "1 or 2 fluorophore selection", "Update configurations", "Update template", "Calculate other values", "Update filter names", "Shutdown", "Shutdown - hard exit", "Search in filters - set parameters", "Search in filters - search", "Search in filters - get xijk", "Search in filters - reget", "Optimize - Sort table", "Get path from search", "Calculate Xijk", "Get spectra from files", "Create graphs", "Reset variables", "Tools - convert image to text", "Tools - create function", "Help - open", "Help - close", "Help - next", "Help - previous", "Help - select menu", "Export data"]
        n304 = call "xijk_array_to_queue.vi"("error in"=w726, "array in"=w724, "queue in"=w725) -> ("error out"=w723:errorcluster)  [unwired: 7 in, 1 out]
        n305 = call "xijk_change_save_location.vi"("error in"=w723, "Settings"=w713) -> ("error out"=w720:errorcluster, "Settings out"=w715:T1)  [unwired: 8 in]
        n306 = local read "Select template"() -> (w718:u16)
        n307 = call "xijk_get_search_table.vi"("template in"=w718, "error in"=w720, "Settings"=w715) -> ("error out"=w719:errorcluster, "Settings out"=w714:T1)  [unwired: 7 in]
        n308 = Unbundle By Name(w714) -> ("search parameters.Paths.Path reget"=w716:path)
        n309 = Unbundle By Name(w714) -> ("search parameters.Paths.Path reget"=w729:path, "search parameters.table for calculation automagic"=w727:i32[])
        n310 = local write "Path reget"(w716) -> ()
        n311 = call "xijk_select_best_filter.vi"("error in"=w719, "calculation table"=w727, "Column Sort Order"=i32[] [22], "file to be analyzed"=w729) -> ("error out"=w721:errorcluster, "sorted output paths table"=w717:string[][])  [unwired: 6 in]
        n312 = call "xijk_search_sorttable_to_paths.vi"("error in"=w721, "sorted output paths table"=w717, "Settings"=w714) -> ("error out"=w722:errorcluster, "Settings out"=w712:T1)  [unwired: 7 in]
      }
      frame "Help - open" {
        n313 = Compound Arithmetic op=OR("Help Templates", "Help Templates 3", "Help Templates 4", "Help Templates 5", "Help Templates 6", "Help Templates 7", "Help Templates 8", "Help Templates 9", FALSE ("value")) -> (w752:bool)
        n314 = Or(x="Help Exciter 2", y="Help Exciter") -> (x .or. y?=w733:bool)
        n315 = Build Array("Button Help", "Help Fluorophore", w733, "Help Filters", "Help Detector", w752, "Help Examples", "Help Eijk", "Help Xijk", "Help Others", "Help Config", "Help Automatized", "Help pictograms") -> (w740:bool[])
        n316 = Boolean Array To Number(Boolean array=w740) -> (number=w739:u32)
        n317 = case shown="False" "Button Help" {
          tunnel: w739 -> [w767 w769]
          tunnel: [w767 w768] -> w738
          frame False {
          }
          frame True {
            n318 = Decrement(x=w769) -> (x-1=w768:u32)
          }
        }
        n319 = To Double Precision Float(number=w738) -> (double precision float=w743:dbl)
        n320 = Logarithm Base 2(1:w743) -> (0:w744:dbl)
        n321 = To Unsigned Long Integer(number=w744) -> (unsigned 32bit integer=w736:u32)
        n322 = call "xijk_set_help_position.vi"("tab in"=w736) -> ("position left out"=w737:i32)  [unwired: 10 in]
        n323 = property on="Tabs wizard" class="TabCtl (strict)"(error in=w763, "Visible"=TRUE, "Value"=w736, "Left"=w737) -> (error out=w764:errorcluster)  [unwired: 1 in, 1 out]
      }
      frame "Help - close" {
        n324 = property on="Tabs wizard" class="TabCtl (strict)"(error in=w771, "Visible"=FALSE) -> (error out=w772:errorcluster)  [unwired: 1 in, 1 out]
      }
      frame "Help - select menu" {
      }
      frame "Help - next" {
        n325 = property on="Tabs wizard" class="TabCtl (strict)"(error in=w788) -> (error out=w789:errorcluster, "Value"=w790:T12)  [unwired: 1 in, 1 out]
        n326 = Increment(x=w790) -> (x+1=w779:T12)
        n327 = call "xijk_set_help_position.vi"("tab in"=w779) -> ("position left out"=w787:i32)  [unwired: 10 in]
        n328 = property on="Tabs wizard" class="TabCtl (strict)"(error in=w789, "Value"=w779, "Left"=w787) -> (error out=w781:errorcluster)  [unwired: 1 in, 1 out]
        n329 = To Long Integer(number=w779) -> (32bit integer=w783:i32)
        n330 = Decrement(x=w783) -> (x-1=w784:i32)
        n331 = property on="Tabs parameters" class="TabCtl (strict)"(error in=w781, "Value"=w784) -> (error out=w786:errorcluster)  [unwired: 1 in, 1 out]
        n332 = Subtract(x=w783, y=7) -> (x-y=w785:i32)
        n333 = property on="Tab results" class="TabCtl (strict)"(error in=w786, "Value"=w785) -> (error out=w780:errorcluster)  [unwired: 1 in, 1 out]
      }
      frame "Help - previous" {
        n334 = property on="Tabs wizard" class="TabCtl (strict)"(error in=w803) -> (error out=w804:errorcluster, "Value"=w798:T12)  [unwired: 1 in, 1 out]
        n335 = Decrement(x=w798) -> (x-1=w796:T12)
        n336 = call "xijk_set_help_position.vi"("tab in"=w796) -> ("position left out"=w802:i32)  [unwired: 10 in]
        n337 = property on="Tabs wizard" class="TabCtl (strict)"(error in=w804, "Value"=w796, "Left"=w802) -> (error out=w793:errorcluster)  [unwired: 1 in, 1 out]
        n338 = To Long Integer(number=w796) -> (32bit integer=w795:i32)
        n339 = Decrement(x=w795) -> (x-1=w797:i32)
        n340 = property on="Tabs parameters" class="TabCtl (strict)"(error in=w793, "Value"=w797) -> (error out=w800:errorcluster)  [unwired: 1 in, 1 out]
        n341 = Subtract(x=w795, y=7) -> (x-y=w799:i32)
        n342 = property on="Tab results" class="TabCtl (strict)"(error in=w800, "Value"=w799) -> (error out=w801:errorcluster)  [unwired: 1 in, 1 out]
      }
      frame "Tools - convert image to text" {
        n343 = call "xijk_image_read.vi"("error in (no error)"=w807, "path in"=path "") -> ("error out"=w808:errorcluster)  [unwired: 8 in, 1 out]
      }
      frame "Tools - create function" {
        n344 = call "xijk_create_function.vi"("error in (no error)"=w811) -> ("error out"=w812:errorcluster)  [unwired: 10 in]
      }
    }
    n345 = case shown="True" w49 {
      frame False {
      }
      frame True {
        n346 = local read "start time"() -> (w63:u32)
        n347 = Tick Count (ms)() -> (millisecond timer value=w64:u32)
        n348 = Subtract(x=w64, y=w63) -> (x-y=w65:u32)
        n349 = To Double Precision Float(number=w65) -> (double precision float=w67:dbl)
        n350 = Divide(x=w67, y=1000.0) -> (x/y=→"Runtime":dbl)
      }
    }
    n351 = case shown="False" w55 {
      frame False {
      }
      frame True {
        n352 = Tick Count (ms)() -> (millisecond timer value=→"start time":u32)
      }
    }
  }
  n353 = while {
    tunnel: w26 -> [w818]
    shift-right: [w816] -> w35
    shift-left: w30 -> [w817]
    stop <- w815 stop-if-true
    n354 = event shown="[22] \"button:create_function\": Value Change" {
      selector: _ -> [_ _ _ _ _ _ _ _ _ _ _ _ _ _ _ _ _ _ _ _ _ _ _]
      dyn-events: _ -> [_ _ _ _ _ _ _ _ _ _ _ _ _ _ _ _ _ _ _ _ _ _ _]
      timeout: _ -> [_ _ _ _ _ _ _ _ _ _ _ _ _ _ _ _ _ _ _ _ _ _ _]
      tunnel: w818 -> [_ w821 w827 w829 w833 w839 w843 w848 w853 w855 w859 w862 w868 w872 w878 w884 w889 _ w894 w898 _ w930 w934]
      tunnel: w817 -> [w819 w820 w825 w830 w835 w838 w844 w846 w852 w854 w861 w864 w867 w871 w877 w883 w888 w892 w896 w900 w901 w929 w932]
      tunnel: [w819 w823 w824 w831 w834 w837 w842 w849 w851 w857 w860 w863 w866 w873 w876 w885 w887 w891 w895 w899 w902 w928 w931] -> w816
      tunnel: [_ _ _ _ _ _ _ _ _ _ _ _ TRUE _ _ _ _ _ _ _ _ _ _] -> w815
      event Timeout {
        n355 = event-data() -> ()  [unwired: 1 in, 2 out]
      }
      event "Extra em filter 2", "Extra em filter 1", "Dichroic filter 2", "Excitation filter 1", "Dichroic filter 1", "Emission filter 1", "Emission filter 2", "Excitation filter 2", "Fluorophore absorption", "Fluorophore emission", "Fluorophore absorption 2", "Fluorophore emission 2", "Light source file", "Quantum efficiency 1", "Quantum efficiency 2", "Molar extinction 1", "Molar extinction 2", "FRET", "Broadness of laser (nm) 1", "Broadness of laser (nm) 2", "Wavelength of laser (nm) 1", "Wavelength of laser (nm) 2", "Detector", "Dual emission by cubes": Value Change {
        w822 = T15[] [enum."Initialise parameters", enum."Initialise paths", enum."Calculate other values", enum."Update filter names", enum."Get spectra from files", enum."Calculate Xijk", enum."Create graphs"] items=["Initialise parameters", "Initialise paths", "Execute", "Hide detector", "Light source selection", "Get example list", "Set Example", "Change portrait / landscape", "Dual band cube", "Save to file", "Load from file", "Set filepaths to boxes", "1 or 2 fluorophore selection", "Update configurations", "Update template", "Calculate other values", "Update filter names", "Shutdown", "Shutdown - hard exit", "Search in filters - set parameters", "Search in filters - search", "Search in filters - get xijk", "Search in filters - reget", "Optimize - Sort table", "Get path from search", "Calculate Xijk", "Get spectra from files", "Create graphs", "Reset variables", "Tools - convert image to text", "Tools - create function", "Help - open", "Help - close", "Help - next", "Help - previous", "Help - select menu", "Export data"]
        n356 = event-data() -> ()  [unwired: 1 in, 5 out]
        n357 = call "xijk_array_to_queue.vi"("error in"=w820, "array in"=w822, "queue in"=w821) -> ("error out"=w823:errorcluster)  [unwired: 7 in, 1 out]
      }
      event "Path reget": Value Change {
        n358 = event-data() -> ()  [unwired: 1 in, 5 out]
        n359 = Enqueue Element(queue=w827, element=event."Initialise paths", error in (no error)=w825) -> (error out=w824:errorcluster)  [unwired: 1 in, 2 out]
      }
      event Value Change {
        w828 = T15[] [enum."Create graphs", enum."Change portrait / landscape"] items=["Initialise parameters", "Initialise paths", "Execute", "Hide detector", "Light source selection", "Get example list", "Set Example", "Change portrait / landscape", "Dual band cube", "Save to file", "Load from file", "Set filepaths to boxes", "1 or 2 fluorophore selection", "Update configurations", "Update template", "Calculate other values", "Update filter names", "Shutdown", "Shutdown - hard exit", "Search in filters - set parameters", "Search in filters - search", "Search in filters - get xijk", "Search in filters - reget", "Optimize - Sort table", "Get path from search", "Calculate Xijk", "Get spectra from files", "Create graphs", "Reset variables", "Tools - convert image to text", "Tools - create function", "Help - open", "Help - close", "Help - next", "Help - previous", "Help - select menu", "Export data"]
        n360 = event-data() -> ()  [unwired: 1 in, 1 out]
        n361 = call "xijk_array_to_queue.vi"("error in"=w830, "array in"=w828, "queue in"=w829) -> ("error out"=w831:errorcluster)  [unwired: 7 in, 1 out]
      }
      event "Number of fluorophores": Value Change {
        w832 = T15[] [enum."1 or 2 fluorophore selection", enum."Initialise parameters"] items=["Initialise parameters", "Initialise paths", "Execute", "Hide detector", "Light source selection", "Get example list", "Set Example", "Change portrait / landscape", "Dual band cube", "Save to file", "Load from file", "Set filepaths to boxes", "1 or 2 fluorophore selection", "Update configurations", "Update template", "Calculate other values", "Update filter names", "Shutdown", "Shutdown - hard exit", "Search in filters - set parameters", "Search in filters - search", "Search in filters - get xijk", "Search in filters - reget", "Optimize - Sort table", "Get path from search", "Calculate Xijk", "Get spectra from files", "Create graphs", "Reset variables", "Tools - convert image to text", "Tools - create function", "Help - open", "Help - close", "Help - next", "Help - previous", "Help - select menu", "Export data"] ("array in")
        n362 = event-data() -> ()  [unwired: 1 in, 1 out]
        n363 = call "xijk_array_to_queue.vi"("error in"=w835, "array in"=w832, "queue in"=w833) -> ("error out"=w834:errorcluster)  [unwired: 7 in, 1 out]
      }
      event "Unknown detector": Value Change {
        w840 = T15[] [enum."Hide detector", enum."Initialise parameters", enum."Update filter names", enum."Get spectra from files", enum."Calculate Xijk", enum."Create graphs"] items=["Initialise parameters", "Initialise paths", "Execute", "Hide detector", "Light source selection", "Get example list", "Set Example", "Change portrait / landscape", "Dual band cube", "Save to file", "Load from file", "Set filepaths to boxes", "1 or 2 fluorophore selection", "Update configurations", "Update template", "Calculate other values", "Update filter names", "Shutdown", "Shutdown - hard exit", "Search in filters - set parameters", "Search in filters - search", "Search in filters - get xijk", "Search in filters - reget", "Optimize - Sort table", "Get path from search", "Calculate Xijk", "Get spectra from files", "Create graphs", "Reset variables", "Tools - convert image to text", "Tools - create function", "Help - open", "Help - close", "Help - next", "Help - previous", "Help - select menu", "Export data"]
        n364 = event-data() -> ("NewVal"=→"hide detector box?":bool)  [unwired: 1 in, 4 out]
        n365 = call "xijk_array_to_queue.vi"("error in"=w838, "array in"=w840, "queue in"=w839) -> ("error out"=w837:errorcluster)  [unwired: 7 in, 1 out]
      }
      event "Light source": Value Change {
        w845 = T15[] [enum."Light source selection", enum."Initialise parameters", enum."Initialise paths", enum."Update filter names", enum."Get spectra from files", enum."Calculate Xijk", enum."Create graphs"] items=["Initialise parameters", "Initialise paths", "Execute", "Hide detector", "Light source selection", "Get example list", "Set Example", "Change portrait / landscape", "Dual band cube", "Save to file", "Load from file", "Set filepaths to boxes", "1 or 2 fluorophore selection", "Update configurations", "Update template", "Calculate other values", "Update filter names", "Shutdown", "Shutdown - hard exit", "Search in filters - set parameters", "Search in filters - search", "Search in filters - get xijk", "Search in filters - reget", "Optimize - Sort table", "Get path from search", "Calculate Xijk", "Get spectra from files", "Create graphs", "Reset variables", "Tools - convert image to text", "Tools - create function", "Help - open", "Help - close", "Help - next", "Help - previous", "Help - select menu", "Export data"]
        n366 = event-data() -> ("NewVal"=→"light source value":u16)  [unwired: 1 in, 4 out]
        n367 = call "xijk_array_to_queue.vi"("error in"=w844, "array in"=w845, "queue in"=w843) -> ("error out"=w842:errorcluster)  [unwired: 7 in, 1 out]
      }
      event "Select template": Value Change {
        w847 = T15[] [enum."Create graphs", enum."Update template", enum."Update configurations", enum."Light source selection", enum."1 or 2 fluorophore selection", enum."Initialise parameters", enum."Initialise paths", enum."Get spectra from files", enum."Calculate Xijk", enum."Create graphs"] items=["Initialise parameters", "Initialise paths", "Execute", "Hide detector", "Light source selection", "Get example list", "Set Example", "Change portrait / landscape", "Dual band cube", "Save to file", "Load from file", "Set filepaths to boxes", "1 or 2 fluorophore selection", "Update configurations", "Update template", "Calculate other values", "Update filter names", "Shutdown", "Shutdown - hard exit", "Search in filters - set parameters", "Search in filters - search", "Search in filters - get xijk", "Search in filters - reget", "Optimize - Sort table", "Get path from search", "Calculate Xijk", "Get spectra from files", "Create graphs", "Reset variables", "Tools - convert image to text", "Tools - create function", "Help - open", "Help - close", "Help - next", "Help - previous", "Help - select menu", "Export data"] ("array in")
        n368 = event-data() -> ()  [unwired: 1 in, 5 out]
        n369 = call "xijk_array_to_queue.vi"("error in"=w846, "array in"=w847, "queue in"=w848) -> ("error out"=w849:errorcluster)  [unwired: 7 in, 1 out]
      }
      event "Examples": Value Change {
        n370 = event-data() -> ()  [unwired: 1 in, 5 out]
        n371 = Enqueue Element(queue=w853, element=event."Set Example", error in (no error)=w852) -> (error out=w851:errorcluster)  [unwired: 1 in, 2 out]
      }
      event "Button save": Value Change {
        w856 = T15[] [enum."Search in filters - set parameters", enum."Save to file"] items=["Initialise parameters", "Initialise paths", "Execute", "Hide detector", "Light source selection", "Get example list", "Set Example", "Change portrait / landscape", "Dual band cube", "Save to file", "Load from file", "Set filepaths to boxes", "1 or 2 fluorophore selection", "Update configurations", "Update template", "Calculate other values", "Update filter names", "Shutdown", "Shutdown - hard exit", "Search in filters - set parameters", "Search in filters - search", "Search in filters - get xijk", "Search in filters - reget", "Optimize - Sort table", "Get path from search", "Calculate Xijk", "Get spectra from files", "Create graphs", "Reset variables", "Tools - convert image to text", "Tools - create function", "Help - open", "Help - close", "Help - next", "Help - previous", "Help - select menu", "Export data"] ("array in")
        n372 = event-data() -> ()  [unwired: 1 in, 5 out]
        n373 = call "xijk_array_to_queue.vi"("error in"=w854, "array in"=w856, "queue in"=w855) -> ("error out"=w857:errorcluster)  [unwired: 7 in, 1 out]
      }
      event "Button load": Value Change {
        n374 = event-data() -> ()  [unwired: 1 in, 5 out]
        n375 = Enqueue Element(queue=w859, element=event."Load from file", error in (no error)=w861) -> (error out=w860:errorcluster)  [unwired: 1 in, 2 out]
      }
      event "Button reset": Value Change {
        n376 = event-data() -> ()  [unwired: 1 in, 5 out]
        n377 = Enqueue Element(queue=w862, element=event."Reset variables", error in (no error)=w864) -> (error out=w863:errorcluster)  [unwired: 1 in, 2 out]
      }
      event "Button stop": Value Change {
        n378 = event-data() -> ()  [unwired: 1 in, 5 out]
        n379 = Enqueue Element At Opposite End(queue=w868, element=event."Shutdown", error in (no error)=w867) -> (error out=w866:errorcluster)  [unwired: 1 in, 2 out]
      }
      event "Button automagic": Value Change {
        w874 = T15[] [enum."Search in filters - set parameters", enum."Search in filters - search", enum."Get path from search"] items=["Initialise parameters", "Initialise paths", "Execute", "Hide detector", "Light source selection", "Get example list", "Set Example", "Change portrait / landscape", "Dual band cube", "Save to file", "Load from file", "Set filepaths to boxes", "1 or 2 fluorophore selection", "Update configurations", "Update template", "Calculate other values", "Update filter names", "Shutdown", "Shutdown - hard exit", "Search in filters - set parameters", "Search in filters - search", "Search in filters - get xijk", "Search in filters - reget", "Optimize - Sort table", "Get path from search", "Calculate Xijk", "Get spectra from files", "Create graphs", "Reset variables", "Tools - convert image to text", "Tools - create function", "Help - open", "Help - close", "Help - next", "Help - previous", "Help - select menu", "Export data"] ("array in")
        n380 = event-data() -> ()  [unwired: 1 in, 5 out]
        n381 = call "xijk_array_to_queue.vi"("error in"=w871, "array in"=w874, "queue in"=w872) -> ("error out"=w873:errorcluster)  [unwired: 7 in, 1 out]
      }
      event "Button Help", "Help pictograms", "Help Examples", "Help Templates 9", "Help Templates 8", "Help Templates 7", "Help Templates 6", "Help Templates 5", "Help Templates 4", "Help Templates 3", "Help Templates", "Help Automatized", "Help Config", "Help Others", "Help Xijk", "Help Eijk", "Help Detector", "Help Filters", "Help Exciter", "Help Fluorophore", "Help Exciter 2": Value Change {
        n382 = event-data() -> ("NewVal"=w879:bool)  [unwired: 1 in, 4 out]
        n383 = case shown="True" w879 {
          tunnel: [event."Help - close" ("element") event."Help - open" ("element")] -> w875
          frame False {
          }
          frame True {
          }
        }
        n384 = Enqueue Element(queue=w878, element=w875, error in (no error)=w877) -> (error out=w876:errorcluster)  [unwired: 1 in, 2 out]
      }
      event "Select result number": Value Change {
        w882 = T15[] [enum."Search in filters - reget", enum."Set filepaths to boxes", enum."Initialise parameters", enum."Initialise paths", enum."Update filter names", enum."Get spectra from files", enum."Calculate Xijk", enum."Create graphs"] items=["Initialise parameters", "Initialise paths", "Execute", "Hide detector", "Light source selection", "Get example list", "Set Example", "Change portrait / landscape", "Dual band cube", "Save to file", "Load from file", "Set filepaths to boxes", "1 or 2 fluorophore selection", "Update configurations", "Update template", "Calculate other values", "Update filter names", "Shutdown", "Shutdown - hard exit", "Search in filters - set parameters", "Search in filters - search", "Search in filters - get xijk", "Search in filters - reget", "Optimize - Sort table", "Get path from search", "Calculate Xijk", "Get spectra from files", "Create graphs", "Reset variables", "Tools - convert image to text", "Tools - create function", "Help - open", "Help - close", "Help - next", "Help - previous", "Help - select menu", "Export data"]
        n385 = event-data() -> ()  [unwired: 1 in, 5 out]
        n386 = call "xijk_array_to_queue.vi"("error in"=w883, "array in"=w882, "queue in"=w884) -> ("error out"=w885:errorcluster)  [unwired: 7 in, 1 out]
      }
      event "Button export": Value Change {
        n387 = event-data() -> ()  [unwired: 1 in, 5 out]
        n388 = Enqueue Element(queue=w889, element=event."Export data", error in (no error)=w888) -> (error out=w887:errorcluster)  [unwired: 1 in, 2 out]
      }
      event "stop wizard 13", "stop wizard 12", "stop wizard 11", "stop wizard 10", "stop wizard 9", "stop wizard 8", "stop wizard 7", "stop wizard 6", "stop wizard 5", "stop wizard 4", "stop wizard 3", "stop wizard 2", "stop wizard 1": Value Change {
        n389 = event-data() -> ()  [unwired: 1 in, 5 out]
        n390 = property on="Button Help" class="Bool (strict)"(error in=w892, "Val(Sgnl)"=FALSE ("Value (Signaling)")) -> (error out=w891:errorcluster)  [unwired: 1 in, 1 out]
      }
      event "Page 12. Previous", "Page 11. Previous", "Page 10. Previous", "Page 9. Previous", "Page 8. Previous", "Page 7. Previous", "Page 6. Previous", "Page 5. Previous", "Page 4. Previous", "Page 3. Previous", "Page 2. Previous", "Page 1. Previous": Value Change {
        n391 = event-data() -> ()  [unwired: 1 in, 5 out]
        n392 = Enqueue Element(queue=w894, element=event."Help - previous", error in (no error)=w896) -> (error out=w895:errorcluster)  [unwired: 1 in, 2 out]
      }
      event "Page 11. Next", "Page 10. Next", "Page 9. Next", "Page 8. Next", "Page 7. Next", "Page 6. Next", "Page 5. Next", "Page 4. Next", "Page 3. Next", "Page 2. Next", "Page 1. Next", "Page 0. Next": Value Change {
        n393 = event-data() -> ()  [unwired: 1 in, 5 out]
        n394 = Enqueue Element(queue=w898, element=event."Help - next", error in (no error)=w900) -> (error out=w899:errorcluster)  [unwired: 1 in, 2 out]
      }
      event Menu Selection (User) {
        n395 = event-data() -> ("ItemTag"=w903:string)  [unwired: 1 in]
        n396 = case shown="\"Reset\"" w903 {
          tunnel: [w904 w905 w907 w910 w913 w916 w919 w922 w925] -> w902
          tunnel: w901 -> [w904 w905 w908 w911 w914 w917 w920 w923 w926]
          frame Default {
          }
          frame "About" {
            n397 = call "xijk_about_dialog.vi"() -> ()  [unwired: 12 in]
          }
          frame "Help" {
            n398 = property on="Button Help" class="Bool (strict)"(error in=w908, "Val(Sgnl)"=TRUE ("Value (Signaling)")) -> (error out=w907:errorcluster)  [unwired: 1 in, 1 out]
          }
          frame "Save" {
            n399 = property on="Button save" class="Bool (strict)"(error in=w911, "Val(Sgnl)"=FALSE ("Value (Signaling)")) -> (error out=w910:errorcluster)  [unwired: 1 in, 1 out]
          }
          frame "Open" {
            n400 = property on="Button load" class="Bool (strict)"(error in=w914, "Val(Sgnl)"=FALSE ("Value (Signaling)")) -> (error out=w913:errorcluster)  [unwired: 1 in, 1 out]
          }
          frame "Export" {
            n401 = property on="Button export" class="Bool (strict)"(error in=w917, "Val(Sgnl)"=FALSE ("Value (Signaling)")) -> (error out=w916:errorcluster)  [unwired: 1 in, 1 out]
          }
          frame "Exit" {
            n402 = property on="Button stop" class="Bool (strict)"(error in=w920, "Val(Sgnl)"=FALSE ("Value (Signaling)")) -> (error out=w919:errorcluster)  [unwired: 1 in, 1 out]
          }
          frame "Search" {
            n403 = property on="Button automagic" class="Bool (strict)"(error in=w923, "Val(Sgnl)"=FALSE ("Value (Signaling)")) -> (error out=w922:errorcluster)  [unwired: 1 in, 1 out]
          }
          frame "Reset" {
            n404 = property on="Button reset" class="Bool (strict)"(error in=w926, "Val(Sgnl)"=FALSE ("Value (Signaling)")) -> (error out=w925:errorcluster)  [unwired: 1 in, 1 out]
          }
        }
      }
      event "button:image_to_text": Value Change {
        n405 = event-data() -> ()  [unwired: 1 in, 1 out]
        n406 = Enqueue Element(queue=w930, element=event."Tools - convert image to text", error in (no error)=w929) -> (error out=w928:errorcluster)  [unwired: 1 in, 2 out]
      }
      event "button:create_function": Value Change {
        n407 = event-data() -> ()  [unwired: 1 in, 1 out]
        n408 = Enqueue Element(queue=w934, element=event."Tools - create function", error in (no error)=w932) -> (error out=w931:errorcluster)  [unwired: 1 in, 2 out]
      }
    }
  }
  n409 = Release Queue(queue=w36, error in (no error)=w34) -> (error out=w33:errorcluster)  [unwired: 1 in, 2 out]
  n410 = Build Array(w33, w35) -> (w3:errorcluster[])
  n411 = Merge Errors(w3) -> (w32:errorcluster)
  n412 = call <vilib>:"General Error Handler.vi"("error in (no error)"=w32) -> ("error out"=w20:errorcluster)  [unwired: 10 in, 4 out]
  n413 = control-ref of="This Application"() -> (w21:refnum<vi>)
  n414 = property class="App"(reference=w21, error in=w20) -> (error out=w19:errorcluster, "App.Kind"=w18:T21)  [unwired: 1 out]
  n415 = case "close executable" shown="\"Run Time System\"" w18 {
    tunnel: w19 -> [_ w935]
    frame Default {
    }
    frame "Run Time System" {
      n416 = control-ref of="This VI"() -> (w936:refnum<vi>)
      n417 = invoke class="VI" method="FP.Close"(reference=w936, error in=w935) -> ()  [unwired: 1 in, 3 out]
    }
  }
